vi "ADQUIRI_adq.vi"() -> ()   [LabVIEW 2019]
doc: "Programa que faz a leitura e a gravação em arquivo TXT de 13 canais provenientes da placa da National Instruments."
uses:
  <vilib>/DAQmx/read.llb/DAQmx Read (Analog 2D DBL NChan NSamp).vi
  <vilib>/Analysis/baseanly.llb/Mean (DBL).vi
  comunicacao.vi
  Aplicacao_atual_global_adq.vi
  <vilib>/DAQmx/configure/timing.llb/DAQmx Timing (Sample Clock).vi
  <vilib>/DAQmx/miscellaneous.llb/DAQmx Fill In Error Info.vi
  <vilib>/Utility/file.llb/Read Delimited Spreadsheet (string).vi
  <vilib>/Utility/file.llb/Write Delimited Spreadsheet (string).vi
  <vilib>/Analysis/NI_AALBase.lvlib
panel:
  out "P1-P2 VERDE":bool
  in  "pos_processamento":bool
  out "comunica funcionando":bool
  in  "Calibração":bool
  in  "COMUNICA":bool
  out "DAQmx Task Name":refnum<k21>
  in  "Visualizar":bool
  out "led viewing":bool
  out "Configuração":string
  in  "Pontos No Gráfico":dbl(knob)=497.5700948522667 scale=0.0..3000.0
  in  "Frequência":dbl=3000.0
  out "Ok":bool
  out "OK2":bool
  out "Ok R":bool
  out "OK2 R":bool
  out "SKM-AI-KF-COR":dbl
  out "SKM-FI-WF":dbl format="%#.2g"
  out "SKM-FIC-KF-COR":dbl format="%#.2g"
  in  "SAIR":bool
  out "JG(m/s)":dbl
  in  "TempoAquisicao":dbl=60.0
  out "JW(m/s)":dbl format="%#.6g"
  out "JK(m/s)":dbl format="%#.6g"
  out "Timer":i32 caption="Elapsed Time (s)"
  in  "COMEÇAR":bool
  out "Quantidade de\narquivos adquiridos":i64
  out "LED adquiri":bool
  out "Aquisição Automática":bool
  out "Linha de Teste":bool
  in  "Tab Control":enum32{"Gráfico", "Matriz"}(tab)
  out "retirando agua_indicador":bool
  in  "Retirando agua(?)":bool
  out "Aplicação":string
  in  "Help":bool
  out "Gráfico":dbl[][](graph)
  out "C1-M corrente":dbl format="%#_4g"
  out "C1-J corrente":dbl format="%#_4g"
  out "C2-M corrente":dbl format="%#_4g"
  out "C2-J corrente":dbl format="%#_4g"
  out "C3-M corrente":dbl format="%#_4g"
  out "C3-J corrente":dbl format="%#_4g"
  out "C4-M corrente":dbl format="%#_4g"
  out "C4-J corrente":dbl format="%#_4g"
  out "P1 corrente":dbl format="%#_4g"
  out "P2 corrente":dbl format="%#_4g"
  out "P3 corrente":dbl format="%#_4g"
  out "P4 corrente":dbl format="%#_4g"
  out "Pfundo corrente":dbl format="%#_4g"
  out "P4(kPa)":dbl format="%#.2g"
  out "P3(kPa)":dbl format="%#.2g"
  out "P2(kPa)":dbl format="%#.2g"
  out "P1(kPa)":dbl format="%#.2g"
  out "Pfundo(kPa)":dbl format="%#.2g"
  out "P4":dbl format="%#_2g"
  out "C4-J":dbl format="%#_2g"
  out "C4-M":dbl format="%#_2g"
  out "C3-J":dbl format="%#_2g"
  out "P3":dbl format="%#_2g"
  out "C3-M":dbl format="%#_2g"
  out "Pfundo":dbl format="%#_2g"
  out "C2-J":dbl format="%#_2g"
  out "P2":dbl format="%#_2g"
  out "C2-M":dbl format="%#_2g"
  out "P1":dbl format="%#_2g"
  out "C1-M":dbl format="%#_2g"
  out "C1-J":dbl format="%#_2g"
  out "Matriz":dbl[][](array[numeric])
  out "Finalizado":bool
  out "Aquisição":bool
  out "Visualização":bool
  out "Comunicação":bool
  in  "SIK-CV-001 2":bool
  in  "SIW-CV-001 2":bool
  in  "ValoresEnviados":T1
  out "SKS-NC-CV-006":bool
  in  "Valores":T2
  out "P1-P2 RED":bool
  out "P2-P3 RED":bool
  out "P3-P4 RED":bool
  out "P34/L [Pa/m]":dbl
  out "P23/L [Pa/m]":dbl
  out "P12/L [Pa/m]":dbl
  out "Valor Teórico[Pa/m]":dbl
  out "P3-P4 VERDE":bool
  out "P2-P3 VERDE":bool
  out "Valvulas":T3
  out "VALORES UDP":string[](array[string])
  out "reference out":refnum<vi>
  out "error out":errorcluster
  in  "SKM-AI-KF_CORIOLI [kg/m³]":dbl
  in  "SKM-FIC-KF_CORIOLI [kg/s]":dbl
  in  "SIW-CV-001":bool
  in  "SIK-CV-001":bool
  in  "Entrada - SKM-FI-WF [CLP]":dbl
  in  "Escala de Calibracao - SKM-FI-WF":cluster{"Escala Max":dbl, "Escala Min":dbl}
  # "m/s"
  # "<- Aquisição"
  # "[Hz]"
  # "Aquisição"
  # "[s]"
  # "m³/s"
  # "m/s"
  # "CHECK-UP"
  # "[s]"
  # "kg/s"
  # "P1, P3 & P4"
  # "m/s"
  # "kg/m³"
  # "P2"
  # "[mA]"
  # "[V]"
  # "[mA]"
  # "[V]"
  # "[mA]"
  # "[V]"
  # "[kPa]"
  # "[mA]"
  # "[V]"
  # "[mA]"
  # "[V]"
  # "[mA]"
  # "[V]"
  # "[kPa]"
  # "[mA]"
  # "[V]"
  # "[mA]"
  # "[V]"
  # "[mA]"
  # "[V]"
  # "[kPa]"
  # "[mA]"
  # "[V]"
  # "[mA]"
  # "[V]"
  # "[mA]"
  # "[V]"
  # "[kPa]"
  # "[mA]"
  # "[V]"
  # "[kPa]"
  # "MIN"
  # "MAX"
  # "P1"
  # "kPa"
  # "P2"
  # "kPa"
  # "P3"
  # "kPa"
  # "P4"
  # "kPa"
  # "Pfundo"
  # "kPa"
  # "Variáveis Selecionadas Para Aquisição"
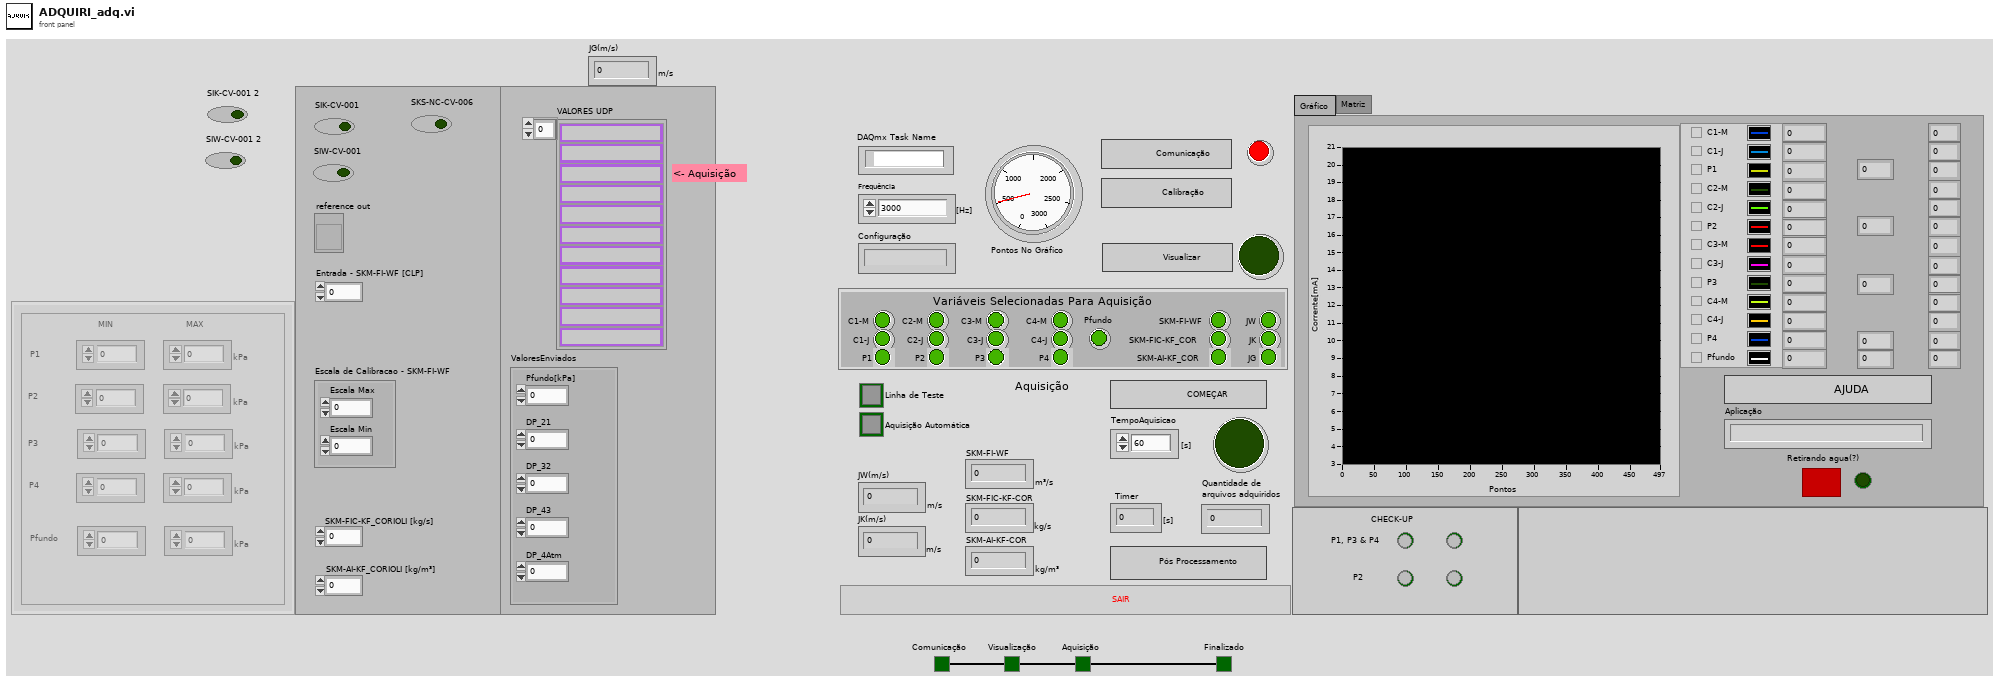
[diagram p1: front panel]
types:
  T1 = cluster{"Pfundo[kPa]":dbl, "DP_21":dbl, "DP_43":dbl, "DP_32":dbl, "DP_4Atm":dbl}
  T2 = cluster{"P1 MIN":i32, "P1 MAX":i32, "P2 MIN":i32, "P2 MAX":i32, "P3 MIN":i32, "P3 MAX":i32, "P4 MIN":i32, "P4 MAX":i32, "Pfu MIN":i32, "Pfu MAX":i32}
  T3 = cluster{"C1-M":bool, "C1-J":bool, "P1":bool, "C2-M":bool, "C2-J":bool, "P2":bool, "C3-M":bool, "C3-J":bool, "P3":bool, "C4-M":bool, "C4-J":bool, "P4":bool, "Pfundo":bool, "JW":bool, "JK":bool, "JG":bool, "SKM-FI-WF":bool, "SKM-FIC-KF_COR":bool, "SKM-AI-KF_COR":bool}
  T4 = enum8{"Enabled", "Disabled", "Disabled and Grayed Out"}
  T5 = enum32{"Invalid", "Standard", "Closed", "Hidden", "Minimized", "Maximized"}
  T6 = enum32{"Bad", "Idle", "Run top level", "Running"}
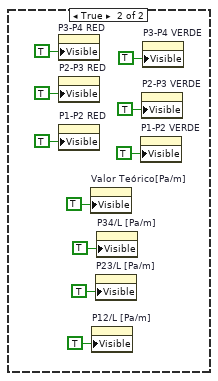
[diagram p3: hidden frame]
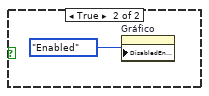
[diagram p5: hidden frame]
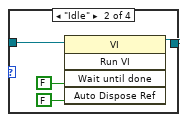
[diagram p6: hidden frame]
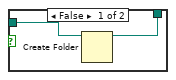
[diagram p9: hidden frame]
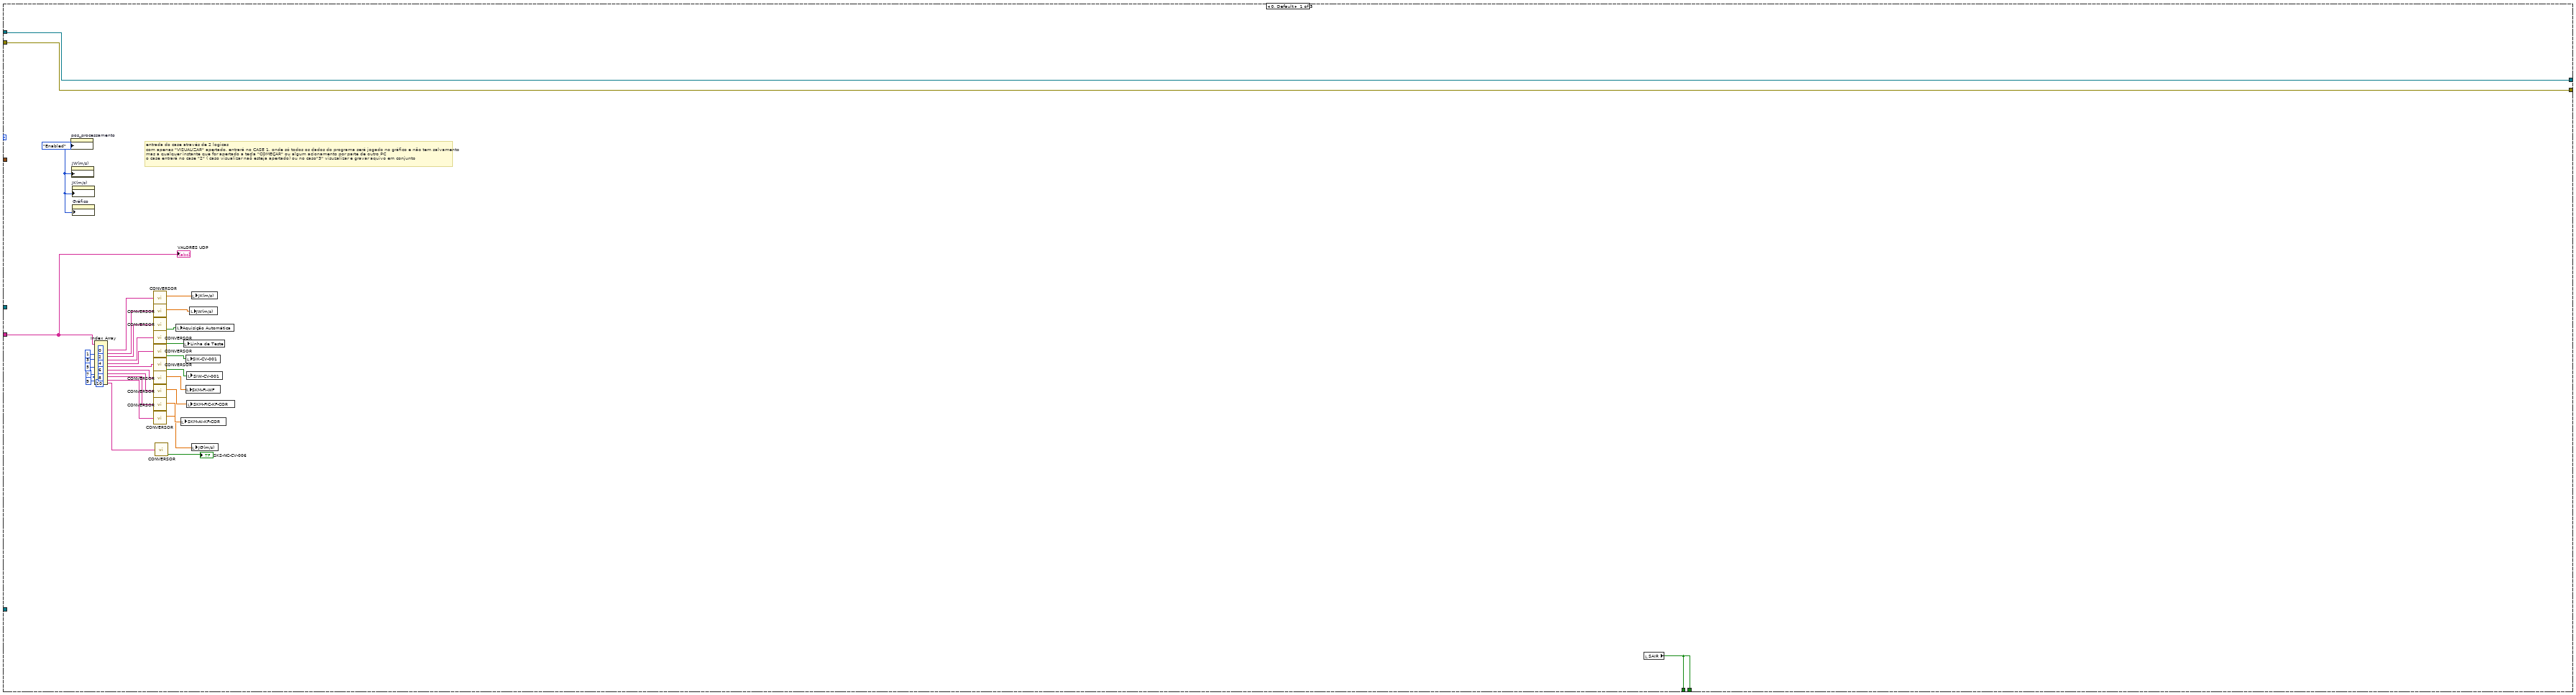
[diagram p11: hidden frame]
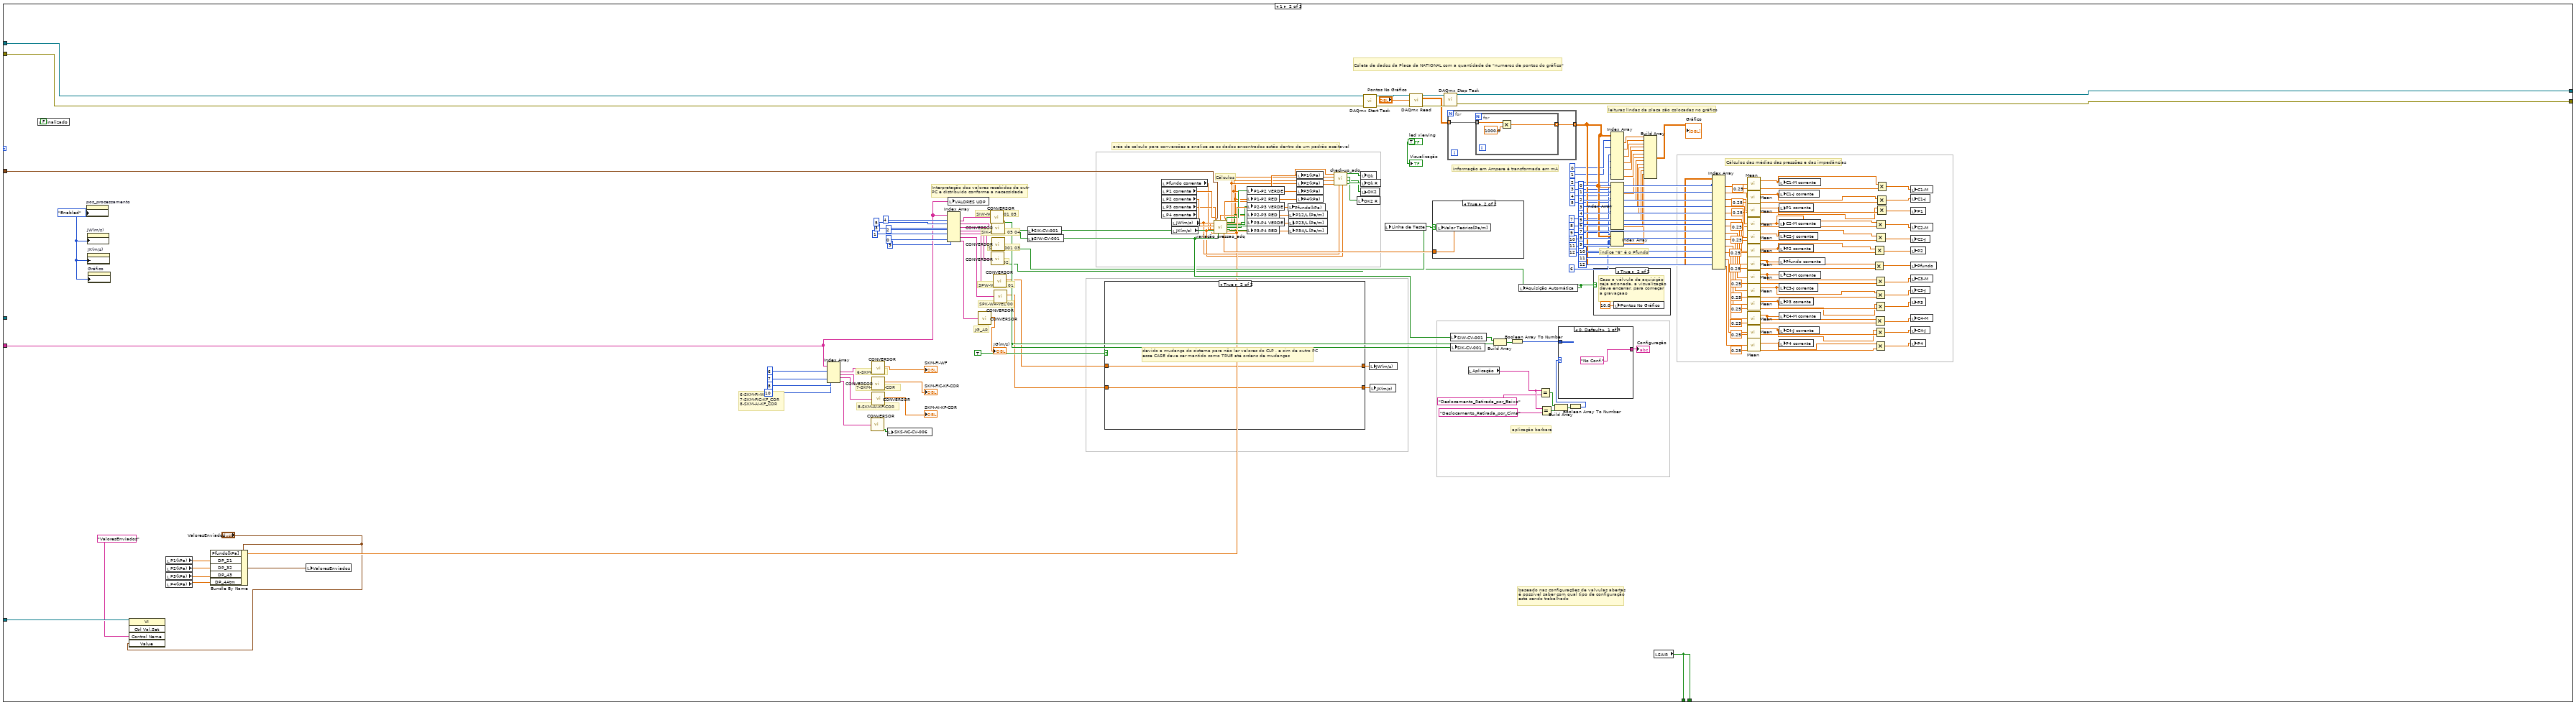
[diagram p12: hidden frame]
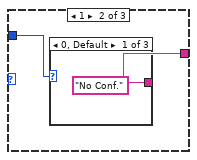
[diagram p13: hidden frame]
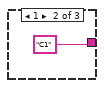
[diagram p14: hidden frame]
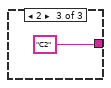
[diagram p15: hidden frame]
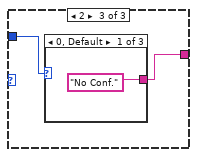
[diagram p16: hidden frame]
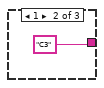
[diagram p17: hidden frame]
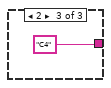
[diagram p18: hidden frame]
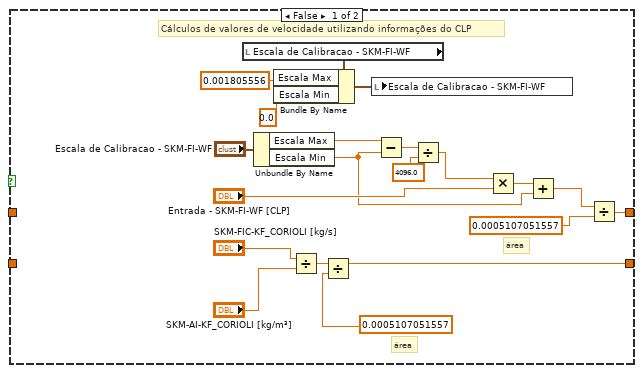
[diagram p19: hidden frame]
diagram:
  # "Abre a VI"
  n1 = property class="VI"("Front Panel.Open"=TRUE ("Front Panel Window:Open")) -> (error out=w1:errorcluster)  [unwired: 2 in, 1 out]
  n2 = flat-sequence {
    tunnel: [w5] -> w3
    tunnel: w1 -> [w4]
    tunnel: w3 -> [w806]
    frame #0 {
      n3 = while {
        shift-right: [w8] -> w5
        shift-left: w4 -> [w7]
        stop <- w6 stop-if-true
        # "Loop responsável\npor manter o \nadquiri rodando\n\nmesmo após uma \naquisição ou \nvisualização dos \ndados\no adquiri não irá\nfechar, e irá \naguardar um novo\ncomando"
        n4 = stacked-sequence {
          tunnel: [w29 _ _ _] -> w8
          tunnel: w7 -> [w29 _ _ _]
          tunnel: [_ _ _ w799] -> w6
          frame #0 {
            w20 = FALSE ("Visualisa")
            w9 = FALSE ("Visualisa")
            w33 = 0.0 ("element")
            # "aplicação barbara"
            # "Nessa parte do cógido, procuramos na aplicação atual, o seu diretório de armazenamento de dados, chamado\n\"DADOS\", cria-o se o mesmo n existir, caso exista, irá retornar a quantidade de arquivos ja adquiridos"
            # "Vi lê as configurações já definidas da aplicação atual e coloca na vairável\n\"VALVULAS\" para facilitar o manuzeio nesse programa"
            # "nessa parte do código , para o ADQUIRI teer acesso a algumas informações do CLP\no computador ADQUIRI evita de comunicar com o CLP para evitar erros futuros, então ele\npega as informações do computador SuperTorre, que é responsável por tratar esses dados\nnessa parte do código, procuramos o diretório UDP e colocamos para rodar o programa\n\"CLIENTE GERAL\" que será responsável por receber as informações do outro PC que contém\no programa\" SERVER GERAL\""
            # "Primeria parte da sequencia  do adquiri, inicia com todas as \nconfigurações e controle em seus estados default\nmatriz de armazenamento com até 17 posições para \narmazenamento de dados e transcrissão para o arquivo txt \nno final da sequencia\npontos no grafico com visualização de 3000 pontos por \nsegundo\ntempo de aquisição inicializado em 30 segundos, mas pode \nser alterado conforme a preferÊncia do usuário\nTimer inicia em 0, que será o tempo atual de aquisição\na configuração da aplicação inicia em default , pois ao longo \ndos acionamento do supervisório, irá saber de qual \nconfiguração se trata\ncontrole de pontos no gráfico encontra ativado\n\nem verde, temos todos os booleanos que necessitam ser\ninicializados em FALSE"
            # "Variáveis que precisam começar com valores iniciais"
            # "indicadores que precisam iniciar desligados"
            n5 = global read "Aplicacao_atual_global_adq.vi" "APLICACAO ATUAL"() -> (w10:string)
            "Aplicação" <- w10
            n6 = flat-sequence {
              frame #0 {
                n7 = global read "comunicacao.vi" "comunicacao"() -> (w55:bool)
                n8 = case shown="False" w55 {
                  frame False {
                    n9 = while {
                      stop <- w56 stop-if-true
                      n10 = One Button Dialog(message="LIGUE O SERVER E \nAPÓS ISSO,\n LIGAR COMUNICAÇÃO", button name ("OK")="OK") -> (true=w56:bool)
                    }
                  }
                  frame True {
                  }
                }
              }
              frame #1 {
                n11 = global read "comunicacao.vi" "comunicacao"() -> (w59:bool)
                n12 = case shown="False" w59 {
                  frame False {
                    n13 = while {
                      stop <- "COMUNICA" stop-if-true
                      n14 = property on="Gráfico" class="WFGraph (strict)"("DisabledEnum"=T4."Disabled and Grayed Out" ("Disabled")) -> ()  [unwired: 2 in, 2 out]
                    }
                  }
                  frame True {
                    n15 = property on="Gráfico" class="WFGraph (strict)"("DisabledEnum"=T4."Enabled" ("Disabled")) -> ()  [unwired: 2 in, 2 out]
                  }
                }
              }
              frame #2 {
                n16 = Current VI's Path() -> (path=w68:path)
                n17 = Strip Path(path=w68) -> (stripped path=w69:path)  [unwired: 1 out]
                n18 = Strip Path(path=w69) -> (stripped path=w70:path)  [unwired: 1 out]
                n19 = Build Path(base path=w70, name or relative path="UDP\\CLIENTE GERAL.vi") -> (appended path=w71:path)
                n20 = Open VI Reference(vi path=w71) -> (vi reference=w64:refnum<vi>)  [unwired: 5 in, 1 out]
                n21 = property class="VI"(reference=w64) -> (reference out=w65:refnum<vi>, "Exec.State"=w66:T6)  [unwired: 1 in, 1 out]
                n22 = case shown="\"Bad\", Default" w66 {
                  tunnel: w65 -> [w72 w74 w77 w78]
                  tunnel: [w72 w73 w77 w78] -> w63
                  frame "Bad", Default {
                  }
                  frame "Idle" {
                    n23 = invoke class="VI" method="Run VI"(reference=w74, "Wait until done"=FALSE ("Wait Until Done"), "Auto Dispose Ref"=FALSE ("Auto Dispose Reference")) -> (reference out=w73:refnum<vi>)  [unwired: 2 in, 4 out]
                  }
                  frame "Run top level" {
                  }
                  frame "Running" {
                  }
                }
                "reference out" <- w63
              }
            }
            n24 = Current VI's Path() -> (path=w28:path)
            n25 = Strip Path(path=w28) -> (stripped path=w27:path)  [unwired: 1 out]
            n26 = Equal?(x=w10, y="Deslocamento_Retirada_por_Baixo") -> (x = y?=w17:bool)
            n27 = Equal?(x=w10, y="Deslocamento_Retirada_por_Cima") -> (x = y?=w16:bool)
            n28 = Or(x=w17, y=w16) -> (x .or. y?=w15:bool)
            n29 = Build Path(base path=w27, name or relative path="PosProcessamento_UDP_NI\\data") -> (appended path=w23:path)
            n30 = property on="Pontos No Gráfico" class="Knob (strict)"("DisabledEnum"=T4."Enabled" ("Disabled")) -> ()  [unwired: 2 in, 2 out]
            n31 = property on="Calibração" class="Bool (strict)"("DisabledEnum"=T4."Enabled" ("Disabled")) -> ()  [unwired: 2 in, 2 out]
            n32 = Initialize Array(w33, w33, 16.0 ("element")) -> (→"Matriz":dbl[][])
            n33 = local write "Configuração"("No Conf." ("Configuration")) -> ()
            n34 = case shown="False" w15 {
              frame False {
                n35 = property on="P3-P4 RED" class="Bool (strict)"("Visible"=FALSE) -> ()  [unwired: 2 in, 2 out]
                n36 = property on="P2-P3 RED" class="Bool (strict)"("Visible"=FALSE) -> ()  [unwired: 2 in, 2 out]
                n37 = property on="P1-P2 RED" class="Bool (strict)"("Visible"=FALSE) -> ()  [unwired: 2 in, 2 out]
                n38 = property on="P1-P2 VERDE" class="Bool (strict)"("Visible"=FALSE) -> ()  [unwired: 2 in, 2 out]
                n39 = property on="P2-P3 VERDE" class="Bool (strict)"("Visible"=FALSE) -> ()  [unwired: 2 in, 2 out]
                n40 = property on="P3-P4 VERDE" class="Bool (strict)"("Visible"=FALSE) -> ()  [unwired: 2 in, 2 out]
                n41 = property on="P12/L [Pa/m]" class="DigNum (strict)"("Visible"=FALSE) -> ()  [unwired: 2 in, 2 out]
                n42 = property on="P23/L [Pa/m]" class="DigNum (strict)"("Visible"=FALSE) -> ()  [unwired: 2 in, 2 out]
                n43 = property on="P34/L [Pa/m]" class="DigNum (strict)"("Visible"=FALSE) -> ()  [unwired: 2 in, 2 out]
                n44 = property on="Valor Teórico[Pa/m]" class="DigNum (strict)"("Visible"=FALSE) -> ()  [unwired: 2 in, 2 out]
              }
              frame True {
                n45 = property on="P3-P4 RED" class="Bool (strict)"("Visible"=TRUE) -> ()  [unwired: 2 in, 2 out]
                n46 = property on="P2-P3 RED" class="Bool (strict)"("Visible"=TRUE) -> ()  [unwired: 2 in, 2 out]
                n47 = property on="P1-P2 RED" class="Bool (strict)"("Visible"=TRUE) -> ()  [unwired: 2 in, 2 out]
                n48 = property on="Valor Teórico[Pa/m]" class="DigNum (strict)"("Visible"=TRUE) -> ()  [unwired: 2 in, 2 out]
                n49 = property on="P12/L [Pa/m]" class="DigNum (strict)"("Visible"=TRUE) -> ()  [unwired: 2 in, 2 out]
                n50 = property on="P23/L [Pa/m]" class="DigNum (strict)"("Visible"=TRUE) -> ()  [unwired: 2 in, 2 out]
                n51 = property on="P34/L [Pa/m]" class="DigNum (strict)"("Visible"=TRUE) -> ()  [unwired: 2 in, 2 out]
                n52 = property on="P1-P2 VERDE" class="Bool (strict)"("Visible"=TRUE) -> ()  [unwired: 2 in, 2 out]
                n53 = property on="P2-P3 VERDE" class="Bool (strict)"("Visible"=TRUE) -> ()  [unwired: 2 in, 2 out]
                n54 = property on="P3-P4 VERDE" class="Bool (strict)"("Visible"=TRUE) -> ()  [unwired: 2 in, 2 out]
              }
            }
            n55 = local write "Timer"(0.0 ("Timer")) -> ()
            n56 = call <vilib>:"Check if File or Folder Exists.vi"("path"=w23) -> ("file or folder exists?"=w26:bool, "dup path"=w25:path)  [unwired: 8 in, 1 out]
            n57 = case shown="True" w26 {
              tunnel: w25 -> [w80 w81]
              tunnel: [w79 w81] -> w24
              frame False {
                n58 = Create Folder(path (use dialog)=w80) -> (created path=w79:path)  [unwired: 2 in, 2 out]
              }
              frame True {
              }
            }
            n59 = File/Directory Info(path=w24) -> (size=w13:i64)  [unwired: 1 in, 6 out]
            n60 = local write "Visualização"(w9) -> ()
            n61 = local write "led viewing"(w9) -> ()
            n62 = local write "LED adquiri"(w9) -> ()
            n63 = local write "Visualizar"(w9) -> ()
            n64 = local write "P1-P2 VERDE"(w9) -> ()
            n65 = local write "P1-P2 RED"(w9) -> ()
            n66 = local write "P2-P3 VERDE"(w9) -> ()
            n67 = local write "P2-P3 RED"(w9) -> ()
            n68 = local write "P3-P4 VERDE"(w9) -> ()
            n69 = local write "P3-P4 RED"(w9) -> ()
            n70 = local write "COMEÇAR"(w9) -> ()
            n71 = local write "Help"(w9) -> ()
            n72 = local write "SAIR"(w9) -> ()
            n73 = local write "Aquisição Automática"(w9) -> ()
            n74 = local write "comunica funcionando"(w9) -> ()
            n75 = local write "Comunicação"(w9) -> ()
            n76 = local write "Aquisição"(w9) -> ()
            n77 = Decrement(x=w13) -> (x-1=→"Quantidade de\narquivos adquiridos":i64)
            n78 = local write "Ok"(w20) -> ()
            n79 = local write "Ok R"(w20) -> ()
            n80 = local write "OK2"(w20) -> ()
            n81 = local write "OK2 R"(w20) -> ()
            n82 = call "leitura_configuracao_valvulas_adq.vi"() -> ("Valvulas"=→"Valvulas":T3)  [unwired: 6 in]
          }
          frame #1 {
            # "nessa etapa do programa, pegamos as referências dessas Vi\n\"LEITURA VALORES CLIENTE\" E \"CLIENTE GERAL\" que JÁ ESTÃO\nRODANDO EM OFF\ncom as refências em mãos, iremos jagá-las para dentro do loop"
            n83 = Current VI's Path() -> (path=w96:path)
            n84 = Current VI's Path() -> (path=w107:path)
            n85 = Strip Path(path=w107) -> (stripped path=w108:path)  [unwired: 1 out]
            n86 = Strip Path(path=w96) -> (stripped path=w90:path)  [unwired: 1 out]
            n87 = Strip Path(path=w108) -> (stripped path=w85:path)  [unwired: 1 out]
            n88 = Build Path(base path=w90, name or relative path="calibracao_adq.vi") -> (appended path=w94:path)
            n89 = Build Path(base path=w85, name or relative path="UDP\\ENVIA VALORES-CLIENTE.vi") -> (appended path=w84:path)
            n90 = Build Path(base path=w85, name or relative path="UDP\\LEITURA VALORES CLIENTE.vi") -> (appended path=w109:path)
            n91 = Build Path(base path=w85, name or relative path="UDP\\CLIENTE GERAL.vi") -> (appended path=w104:path)
            n92 = Open VI Reference(vi path=w84) -> (vi reference=w82:refnum<vi>)  [unwired: 5 in, 1 out]
            n93 = Open VI Reference(vi path=w94, error in (no error)=errorcluster {"status"=FALSE, "code"=0, "source"=""}) -> (vi reference=w93:refnum<vi>, error out=w92:errorcluster)  [unwired: 4 in]
            n94 = Open VI Reference(vi path=w109) -> (vi reference=w105:refnum<vi>)  [unwired: 5 in, 1 out]
            n95 = Open VI Reference(vi path=w104) -> (vi reference=w102:refnum<vi>)  [unwired: 5 in, 1 out]
            n96 = invoke class="VI" method="Run VI"(reference=w93, error in=w92, "Wait until done"=FALSE ("Wait Until Done"), "Auto Dispose Ref"=TRUE ("Auto Dispose Reference")) -> (reference out=w98:refnum<vi>, error out=w97:errorcluster)  [unwired: 1 in, 3 out]
            n97 = invoke class="VI" method="Ctrl Val.Get"(reference=w98, error in=w97, "Control Name"="Valores") -> (reference out=w88:refnum<vi>, error out=w87:errorcluster, "Get Control Value Variant"=w86:variant)  [unwired: 1 in, 1 out]
            n98 = while {
              tunnel: w105 -> [w123]
              tunnel: w102 -> [w146]
              shift-right: [w136] -> w89
              shift-left: w88 -> [w132]
              shift-right: [w135] -> _
              shift-left: w87 -> [w133]
              shift-right: [w131] -> _
              shift-left: w86 -> [w134]
              tunnel: w82 -> [w124]
              stop <- w159 stop-if-true
              w121 = refnum<k21> "ADQUIRE" ("DAQmx Task Name")
              w120 = 10123 items=["Finite Samples"=10178, "Continuous Samples"=10123, "Hardware Timed Single Point"=12522] ("sample mode")
              w111 = FALSE ("visu led")
              # "Parte de comunicação com a placa da NATIONAL\nINSTRUMENTS\nno módulo de comunicação chamado DAQmx\nselecionamos o tipo \"continuous SAMPLES\" para a\ncoleta de amostras contínuas\ntambém entramos com o nome de TASK chamado\nADQUIRE, que já contém informações de leitura \njá pré programadas\nFrequência padrão de 3000Hz"
              # "10"
              # "9"
              # "8"
              # "7"
              # "6"
              # "5"
              # "4"
              # "3"
              # "2"
              # "1"
              # "0"
              # "acionamento automático recebido de outro\nPC"
              # "Default dos botões"
              # "Caso as configurações não desejam\nincluir alguma velocidade na aquisição\na mesma será desabilitada"
              # "Coleta os valores das variáveis enviadas abaixo\nos valores são devolvidos na mesma ordem"
              # "Envia para o programa de comunicação com o outro computador\numa lista de nomes de variáveis que o ADQUIRE nessecita \nos nomes precisam ser enviados em array de STRING para o funcionamento\ndo programa de comunicação."
              # "ADQ 02"
              n99 = local read "Valvulas"() -> (w150:T3)
              n100 = local write "Ok R"(w111) -> ()
              n101 = local write "Visualização"(w111) -> ()
              n102 = local write "led viewing"(w111) -> ()
              n103 = local write "OK2"(w111) -> ()
              n104 = local write "OK2 R"(w111) -> ()
              n105 = local write "Ok"(w111) -> ()
              n106 = case shown="True" "Help" {
                frame False {
                  # "Botão Help destinado a abrir documentos e pesquisas relacionadas\nele também abre uma janela explicando sucintamente o objetivo do \nprograma ADQUIRE"
                }
                frame True {
                  n107 = stacked-sequence {
                    frame #0 {
                      n108 = Current VI's Path() -> (path=w741:path)
                      n109 = Current VI's Path() -> (path=w735:path)
                      n110 = Strip Path(path=w741) -> (stripped path=w740:path)  [unwired: 1 out]
                      n111 = Strip Path(path=w735) -> (stripped path=w734:path)  [unwired: 1 out]
                      n112 = Build Path(base path=w740, name or relative path="Help_difinicao_adq.vi") -> (appended path=w738:path)
                      n113 = Build Path(base path=w734, name or relative path="help_pdfs_adq.vi") -> (appended path=w732:path)
                      n114 = Open VI Reference(vi path=w738) -> (vi reference=w745:refnum<vi>, error out=w744:errorcluster)  [unwired: 5 in]
                      n115 = Open VI Reference(vi path=w732) -> (vi reference=w743:refnum<vi>, error out=w742:errorcluster)  [unwired: 5 in]
                      n116 = invoke class="VI" method="Run VI"(reference=w745, error in=w744, "Wait until done"=FALSE ("Wait Until Done"), "Auto Dispose Ref"=FALSE ("Auto Dispose Reference")) -> ()  [unwired: 1 in, 5 out]
                      n117 = invoke class="VI" method="Run VI"(reference=w743, error in=w742, "Wait until done"=FALSE ("Wait Until Done"), "Auto Dispose Ref"=FALSE ("Auto Dispose Reference")) -> ()  [unwired: 1 in, 5 out]
                    }
                    frame #1 {
                      n118 = local write "Help"(FALSE ("Help")) -> ()
                    }
                  }
                }
              }
              n119 = Unbundle By Name(w150) -> ("JW"=w151:bool, "JK"=w152:bool, "JG"=w153:bool)
              n120 = case shown="True" w151 {
                frame False {
                  n121 = property on="JW(m/s)" class="DigNum (strict)"("DisabledEnum"=T4."Disabled and Grayed Out" ("Disabled")) -> ()  [unwired: 2 in, 2 out]
                }
                frame True {
                  n122 = property on="JW(m/s)" class="DigNum (strict)"("DisabledEnum"=T4."Enabled" ("Disabled")) -> ()  [unwired: 2 in, 2 out]
                }
              }
              n123 = case shown="True" w152 {
                frame False {
                  n124 = property on="JK(m/s)" class="DigNum (strict)"("DisabledEnum"=T4."Disabled and Grayed Out" ("Disabled")) -> ()  [unwired: 2 in, 2 out]
                }
                frame True {
                  n125 = property on="JK(m/s)" class="DigNum (strict)"("DisabledEnum"=T4."Enabled" ("Disabled")) -> ()  [unwired: 2 in, 2 out]
                }
              }
              n126 = case shown="True" w153 {
                frame False {
                  n127 = property on="JG(m/s)" class="DigNum (strict)"("DisabledEnum"=T4."Disabled and Grayed Out" ("Disabled")) -> ()  [unwired: 2 in, 2 out]
                }
                frame True {
                  n128 = property on="JG(m/s)" class="DigNum (strict)"("DisabledEnum"=T4."Enabled" ("Disabled")) -> ()  [unwired: 2 in, 2 out]
                }
              }
              n129 = case shown="False" "Calibração" {
                tunnel: [w705 w713] -> w136
                tunnel: [w706 w712] -> w135
                tunnel: [w707 w711] -> w131
                tunnel: w132 -> [w704 w710]
                tunnel: w133 -> [w703 w709]
                tunnel: w134 -> [_ _]
                frame False {
                  n130 = invoke class="VI" method="Ctrl Val.Get"(reference=w704, error in=w703, "Control Name"="Valores") -> (reference out=w705:refnum<vi>, error out=w706:errorcluster, "Get Control Value Variant"=w707:variant)  [unwired: 1 in, 1 out]
                }
                frame True {
                  n131 = stacked-sequence {
                    tunnel: [w718 _] -> w713
                    tunnel: [w717 _] -> w712
                    tunnel: [w716 _] -> w711
                    tunnel: w710 -> [w715 _]
                    tunnel: w709 -> [w714 _]
                    frame #0 {
                      n132 = invoke class="VI" method="FP.Open"(reference=w715, error in=w714, "State"=T5."Standard") -> (reference out=w720:refnum<vi>, error out=w719:errorcluster)  [unwired: 2 in, 3 out]
                      n133 = invoke class="VI" method="Ctrl Val.Get"(reference=w720, error in=w719, "Control Name"="Valores") -> (reference out=w718:refnum<vi>, error out=w717:errorcluster, "Get Control Value Variant"=w716:variant)  [unwired: 1 in, 1 out]
                    }
                    frame #1 {
                      n134 = local write "Calibração"(FALSE ("Calibração")) -> ()
                    }
                  }
                }
              }
              n135 = invoke class="VI" method="Ctrl Val.Get"(reference=w123, "Control Name"="VALORES") -> ("Get Control Value Variant"=w149:variant)  [unwired: 2 in, 3 out]
              n136 = property on="Gráfico" class="WFGraph (strict)"("DisabledEnum"=T4."Enabled" ("Disabled")) -> ()  [unwired: 2 in, 2 out]
              n137 = Variant To Data(type=string[] [] ("Array"), Variant=w149) -> (data=w128:string[])  [unwired: 1 in, 1 out]
              n138 = To Variant(anything=string[] ["JK", "JW", "ADQ", "SIT-NC-CV-001", "SIK-NC-CV-001", "SIW-NC-CV-001", "SKM-FI-WF", "SKM-FIC-KF_COR", "SKM-AI-KF_COR", "JG", "SKS-NC-CV-006"] ("NOMES")) -> (Variant=w141:variant)
              n139 = case shown="True" "pos_processamento" {
                frame False {
                }
                frame True {
                  n140 = Current VI's Path() -> (path=w169:path)
                  n141 = Strip Path(path=w169) -> (stripped path=w170:path)  [unwired: 1 out]
                  n142 = Build Path(base path=w170, name or relative path="PosProcessamento_UDP_NI\\main_PosProcessamento_UDP_NI.vi") -> (appended path=w171:path)
                  n143 = Open VI Reference(vi path=w171) -> (vi reference=w162:refnum<vi>)  [unwired: 5 in, 1 out]
                  n144 = invoke class="VI" method="FP.Open"(reference=w162, "Activate"=TRUE ("Activate?"), "State"=T5."Standard") -> (reference out=w165:refnum<vi>)  [unwired: 2 in, 4 out]
                  n145 = invoke class="VI" method="Run VI"(reference=w165, "Wait until done"=FALSE ("Wait Until Done")) -> (reference out=w166:refnum<vi>)  [unwired: 3 in, 4 out]
                  n146 = Close Reference(reference=w166) -> ()  [unwired: 1 in, 1 out]
                }
              }
              n147 = invoke class="VI" method="Ctrl Val.Set"(reference=w146, "Control Name"="NOMES", "Value"=w141) -> ()  [unwired: 2 in, 5 out]
              n148 = Index Array(array=w128, index=2) -> (element=w144:string)
              n149 = call "CONVERSOR.vi"("String"=w144) -> ("boolean"=w143:bool)  [unwired: 6 in, 3 out]
              "Aquisição Automática" <- w143
              n150 = Not Equal?(x=w128, y="") -> (x != y?=w127:bool[])
              n151 = Get Variant Attribute(Variant=w131, name="Valores") -> ()  [unwired: 2 in, 4 out]
              n152 = Variant To Data(type="Valores", Variant=w131) -> (data=w129:T2)  [unwired: 1 in, 1 out]
              n153 = Index Array(array=w127, index=0) -> (element=→"comunica funcionando" →"Comunicação":bool)
              n154 = local write "Valores"(w129) -> ()
              n155 = Or(x="COMEÇAR", y=w143) -> (x .or. y?=w156:bool)
              n156 = Build Array("Visualizar", w156) -> (w161:bool[])
              n157 = Boolean Array To Number(Boolean array=w161) -> (number=w160:u32)
              n158 = call-poly <vilib>:"DAQmx Timing.vi"("task/channels in"=w121, "sample mode"=w120, "rate"="Frequência", "source"=tag "OnboardClock") -> ("task out"=w118:refnum<k21>, "error out"=w117:errorcluster)  [unwired: 10 in]
              n159 = case shown="2, 3" w160 {
                tunnel: [w173 w239 w449] -> w158
                tunnel: [w173 w239 w448] -> w157
                tunnel: w128 -> [w207 w313 w447]
                tunnel: w118 -> [w209 w303 _]
                tunnel: w117 -> [w208 w302 _]
                tunnel: [w209 w301 w443] -> w115
                tunnel: [w208 w300 w444] -> w114
                tunnel: w129 -> [_ w257 w446]
                tunnel: w124 -> [_ w244 w445]
                tunnel: w123 -> [_ _ w442]
                frame 0, Default {
                  w172 = T4."Enabled" ("Disabled")
                  # "entrada do case através de 2 logicas\ncom apenas \"VISUALIZAR\" apertado, entrará no CASE 1, onde só todos os dados do programa será jogado no gráfico e não tem salvamento\nmas a qualquer instante que for apertado a tecla \"COMEÇAR\" ou algum acionamento por parte de outro PC\no case entrará no case \"2\" ( caso visualizar naõ esteja apertado) ou no caso\"3\" visuzalizar e gravar aquivo em conjunto"
                  n160 = property on="pos_processamento" class="Bool"("DisabledEnum"=w172) -> ()  [unwired: 2 in, 2 out]
                  n161 = property on="JW(m/s)" class="DigNum (strict)"("DisabledEnum"=w172) -> ()  [unwired: 2 in, 2 out]
                  n162 = property on="JK(m/s)" class="DigNum (strict)"("DisabledEnum"=w172) -> ()  [unwired: 2 in, 2 out]
                  n163 = property on="Gráfico" class="WFGraph (strict)"("DisabledEnum"=w172) -> ()  [unwired: 2 in, 2 out]
                  n164 = Index Array(array=w207, index #1=0 ("index"), index #2=1 ("index"), index #3=2 ("index"), index #4=3 ("index"), index #5=4 ("index"), index #6=5 ("index"), index #7=6 ("index"), index #8=7 ("index"), index #9=8 ("index"), index #10=9 ("index"), index #11=10 ("index")) -> (element #1=w196:string, element #2=w195:string, element #3=w194:string, element #4=w193:string, element #5=w192:string, element #6=w191:string, element #7=w190:string, element #8=w189:string, element #9=w188:string, element #10=w187:string, element #11=w176:string)
                  n165 = call "CONVERSOR.vi"("String"=w196) -> ("float"=w186:dbl)  [unwired: 6 in, 3 out]
                  n166 = call "CONVERSOR.vi"("String"=w195) -> ("float"=w185:dbl)  [unwired: 6 in, 3 out]
                  n167 = call "CONVERSOR.vi"("String"=w194) -> ("boolean"=w184:bool)  [unwired: 6 in, 3 out]
                  n168 = call "CONVERSOR.vi"("String"=w193) -> ("boolean"=w183:bool)  [unwired: 6 in, 3 out]
                  n169 = call "CONVERSOR.vi"("String"=w192) -> ("boolean"=w182:bool)  [unwired: 6 in, 3 out]
                  n170 = call "CONVERSOR.vi"("String"=w191) -> ("boolean"=w181:bool)  [unwired: 6 in, 3 out]
                  n171 = call "CONVERSOR.vi"("String"=w190) -> ("float"=w180:dbl)  [unwired: 6 in, 3 out]
                  n172 = call "CONVERSOR.vi"("String"=w189) -> ("float"=w179:dbl)  [unwired: 6 in, 3 out]
                  n173 = call "CONVERSOR.vi"("String"=w188) -> ("float"=w178:dbl)  [unwired: 6 in, 3 out]
                  n174 = call "CONVERSOR.vi"("String"=w187) -> ("float"=w177:dbl)  [unwired: 6 in, 3 out]
                  n175 = call "CONVERSOR.vi"("String"=w176) -> ("boolean"=→"SKS-NC-CV-006":bool)  [unwired: 6 in, 3 out]
                  n176 = local write "Aquisição Automática"(w184) -> ()
                  n177 = local write "SKM-AI-KF-COR"(w178) -> ()
                  n178 = local write "Linha de Teste"(w183) -> ()
                  n179 = local write "SKM-FI-WF"(w180) -> ()
                  n180 = local write "SIK-CV-001"(w182) -> ()
                  n181 = local write "SIW-CV-001"(w181) -> ()
                  n182 = local write "SKM-FIC-KF-COR"(w179) -> ()
                  n183 = local write "JW(m/s)"(w185) -> ()
                  n184 = local write "JK(m/s)"(w186) -> ()
                  n185 = local write "JG(m/s)"(w177) -> ()
                  n186 = local read "SAIR"() -> (w173:bool)
                  "VALORES UDP" <- w207
                }
                frame 1 {
                  w238 = T4."Enabled" ("Disabled")
                  w241 = TRUE ("visu led")
                  # "Cálculos"
                  # "aplicação barbara"
                  # "JG_AR"
                  # "6-SKM-FI-WF"
                  # "7-SKM-FIC-KF-COR"
                  # "8-SKM-AI-KF-COR"
                  # "6-SKM-FI-WF\n7-SKM-FIC-KF_COR\n8-SKM-AI-KF_COR"
                  # "indice \"6\" é o Pfundo"
                  # "leituras lindas da placa são colocadas no gráfico"
                  # "baseado nas configurações de valvulas abertas\né possível saber com qual tipo de configuração \nestá sendo trabalhado"
                  # "aréa de calculo para conversões e analise se os dados encontrados estão dentro de um padrão aceitavel"
                  # "Interpretação dos valores recebidos de outr\nPC e distribuido conforme a necessidade"
                  # "informação em Ampere é transformada em mA"
                  # "Coleta de dados da Placa da NATIONAL com a quantidade de \"numeros de pontos do gráfico\""
                  # "ADQ 02"
                  # "SIW-NC-CV-001 05"
                  # "SIK-CV-001 05 04"
                  # "SIT-CV-001 03"
                  # "SPW-WR-VEL 01"
                  # "SPK-WR-VEL 00"
                  # "Cálculos das médias das pressões e das impedâncias"
                  n187 = local write "Finalizado"(FALSE ("Finalizado")) -> ()
                  n188 = property on="pos_processamento" class="Bool"("DisabledEnum"=w238) -> ()  [unwired: 2 in, 2 out]
                  n189 = property on="JW(m/s)" class="DigNum (strict)"("DisabledEnum"=w238) -> ()  [unwired: 2 in, 2 out]
                  n190 = property on="JK(m/s)" class="DigNum (strict)"("DisabledEnum"=w238) -> ()  [unwired: 2 in, 2 out]
                  n191 = property on="Gráfico" class="WFGraph (strict)"("DisabledEnum"=w238) -> ()  [unwired: 2 in, 2 out]
                  n192 = invoke class="VI" method="Ctrl Val.Set"(reference=w244, "Control Name"="ValoresEnviados", "Value"="ValoresEnviados") -> ()  [unwired: 2 in, 5 out]
                  n193 = local read "P1(kPa)"() -> (w213:dbl)
                  n194 = local read "P2(kPa)"() -> (w212:dbl)
                  n195 = local read "P3(kPa)"() -> (w211:dbl)
                  n196 = local read "P4(kPa)"() -> (w210:dbl)
                  n197 = Index Array(array=w313, index #1=6 ("index"), index #2=7 ("index"), index #3=8 ("index"), index #4=10 ("index")) -> (element #1=w309:string, element #2=w308:string, element #3=w307:string, element #4=w255:string)
                  n198 = call "CONVERSOR.vi"("String"=w255) -> ("boolean"=w254:bool)  [unwired: 6 in, 3 out]
                  n199 = call "CONVERSOR.vi"("String"=w308) -> ("float"=→"SKM-FIC-KF-COR":dbl)  [unwired: 6 in, 3 out]
                  n200 = call "CONVERSOR.vi"("String"=w309) -> ("float"=→"SKM-FI-WF":dbl)  [unwired: 6 in, 3 out]
                  n201 = call "CONVERSOR.vi"("String"=w307) -> ("float"=→"SKM-AI-KF-COR":dbl)  [unwired: 6 in, 3 out]
                  n202 = local write "SKS-NC-CV-006"(w254) -> ()
                  n203 = Index Array(array=w313, index #1=4 ("index"), index #2=5 ("index"), index #3=3 ("index"), index #4=2 ("index"), index #5=1 ("index"), index #6=0 ("index"), index #7=9 ("index")) -> (element #1=w330:string, element #2=w329:string, element #3=w326:string, element #4=w322:string, element #5=w318:string, element #6=w315:string, element #7=w298:string)
                  n204 = local write "VALORES UDP"(w313) -> ()
                  n205 = call "CONVERSOR.vi"("String"=w298) -> ("float"=→"JG(m/s)":dbl)  [unwired: 6 in, 3 out]
                  n206 = call "CONVERSOR.vi"("String"=w330) -> ("boolean"=w324:bool)  [unwired: 6 in, 3 out]
                  n207 = call "CONVERSOR.vi"("String"=w322) -> ("boolean"=w321:bool)  [unwired: 6 in, 3 out]
                  n208 = call "CONVERSOR.vi"("String"=w329) -> ("boolean"=w328:bool)  [unwired: 6 in, 3 out]
                  n209 = call "CONVERSOR.vi"("String"=w326) -> ("boolean"=w325:bool)  [unwired: 6 in, 3 out]
                  n210 = call "CONVERSOR.vi"("String"=w318) -> ("float"=w317:dbl)  [unwired: 6 in, 3 out]
                  n211 = call "CONVERSOR.vi"("String"=w315) -> ("float"=w314:dbl)  [unwired: 6 in, 3 out]
                  n212 = local write "SIK-CV-001"(w324) -> ()
                  n213 = local write "SIW-CV-001"(w328) -> ()
                  n214 = case shown="True" TRUE {
                    tunnel: [w411 w430] -> w387
                    tunnel: [w410 w431] -> w386
                    tunnel: w317 -> [_ w431]
                    tunnel: w314 -> [_ w430]
                    frame False {
                      # "Cálculos de valores de velocidade utilizando informações do CLP"
                      # "área"
                      # "área"
                      n215 = local read "Escala de Calibracao - SKM-FI-WF"() -> (w417:cluster{"Escala Max":dbl, "Escala Min":dbl})
                      n216 = Unbundle By Name("Escala de Calibracao - SKM-FI-WF") -> ("Escala Max"=w420:dbl, "Escala Min"=w419:dbl)
                      n217 = Bundle By Name(cluster=w417, "Escala Max"=0.001805556, "Escala Min"=0.0 ("Escala Max")) -> (w418:cluster{"Escala Max":dbl, "Escala Min":dbl})
                      n218 = Divide(x="SKM-FIC-KF_CORIOLI [kg/s]", y="SKM-AI-KF_CORIOLI [kg/m³]") -> (x/y=w429:dbl)
                      n219 = Divide(x=w429, y=0.0005107051557) -> (x/y=w411:dbl)
                      n220 = local write "Escala de Calibracao - SKM-FI-WF"(w418) -> ()
                      n221 = Subtract(x=w420, y=w419) -> (x-y=w421:dbl)
                      n222 = Divide(x=w421, y=4096.0) -> (x/y=w422:dbl)
                      n223 = Multiply(x=w422, y="Entrada - SKM-FI-WF [CLP]") -> (x*y=w423:dbl)
                      n224 = Add(x=w423, y=w419) -> (x+y=w426:dbl)
                      n225 = Divide(x=w426, y=0.0005107051557) -> (x/y=w410:dbl)
                    }
                    frame True {
                      # "devido a mudança do sistema para não ler valores do CLP , e sim de outro PC\nesse CASE deve ser mantido como TRUE até ordens de mudanças"
                    }
                  }
                  n226 = local read "Pfundo corrente"() -> (w224:dbl)
                  n227 = local read "P1 corrente"() -> (w237:dbl)
                  n228 = local read "P2 corrente"() -> (w236:dbl)
                  n229 = local read "P3 corrente"() -> (w235:dbl)
                  n230 = local read "P4 corrente"() -> (w228:dbl)
                  n231 = local read "JW(m/s)"() -> (w215:dbl)
                  n232 = local read "JK(m/s)"() -> (w214:dbl)
                  n233 = call "variação_pressao_adq.vi"("P1(mA)"=w237, "P2(mA)"=w236, "P3(mA)"=w235, "P4(mA)"=w228, "PFUNDO(mA)"=w224, "JW(m/s)"=w215, "JK(m/s)"=w214, "Valores"=w257, "SIK-CV-001"=w324, "SIW-CV-001"=w328) -> ("P12/L12"=w229:dbl, "P34/L34"=w231:dbl, "P23/L23"=w230:dbl, "P2(kPa)"=w218:dbl, "VALOR TEORICO"=w391:dbl, "P3(kPa)"=w217:dbl, "P1(kPa)"=w219:dbl, "P4(kPa)"=w216:dbl, "P1-P2G"=w234:bool, "P2-P3R"=w225:bool, "P2-P3G"=w233:bool, "P1-P2R"=w227:bool, "P3-P4G"=w232:bool, "P3-P4R"=w226:bool, "PFUNDO(kPa)"=w245:dbl)  [unwired: 3 in]
                  n234 = Bundle By Name(cluster="ValoresEnviados", "Pfundo[kPa]"=w245, "DP_21"=w213, "DP_32"=w212, "DP_43"=w211, "DP_4Atm"=w210) -> (w246:T1)
                  n235 = local write "ValoresEnviados"(w246) -> ()
                  n236 = local write "P1-P2 VERDE"(w234) -> ()
                  n237 = local write "P1-P2 RED"(w227) -> ()
                  n238 = local write "P2-P3 VERDE"(w233) -> ()
                  n239 = local write "P2-P3 RED"(w225) -> ()
                  n240 = local write "P3-P4 VERDE"(w232) -> ()
                  n241 = local write "P3-P4 RED"(w226) -> ()
                  n242 = local write "Pfundo(kPa)"(w245) -> ()
                  n243 = local write "P12/L [Pa/m]"(w229) -> ()
                  n244 = local write "P23/L [Pa/m]"(w230) -> ()
                  n245 = local write "P34/L [Pa/m]"(w231) -> ()
                  n246 = local write "P1(kPa)"(w219) -> ()
                  n247 = local write "P2(kPa)"(w218) -> ()
                  n248 = local write "P3(kPa)"(w217) -> ()
                  n249 = local write "P4(kPa)"(w216) -> ()
                  n250 = call "check-up_adq.vi"("JK(m/s)"=w214, "JW(m/s)"=w215, "P4(kPa)"=w216, "P3(kPa)"=w217, "P2(kPa)"=w218, "P1(kPa)"=w219) -> ("OK 2 R"=w220:bool, "OK 2 G"=w221:bool, "OK RED"=w222:bool, "OK G"=w223:bool)  [unwired: 2 in]
                  n251 = local write "OK2 R"(w220) -> ()
                  n252 = local write "Ok"(w223) -> ()
                  n253 = local write "Ok R"(w222) -> ()
                  n254 = local write "OK2"(w221) -> ()
                  n255 = call <vilib>:"DAQmx Start Task.vi"("task/channels in"=w303, "error in"=w302) -> ("task out"=w398:refnum<k21>, "error out"=w397:errorcluster)  [unwired: 12 in]
                  n256 = local write "JW(m/s)"(w386) -> ()
                  n257 = local write "JK(m/s)"(w387) -> ()
                  n258 = local write "Linha de Teste"(w325) -> ()
                  n259 = call-poly <vilib>:"DAQmx Read.vi"("task/channels in"=w398, "number of samples per channel"="Pontos No Gráfico", "error in"=w397) -> ("task out"=w396:refnum<k21>, "data"=w394:dbl[][], "error out"=w395:errorcluster)  [unwired: 10 in]
                  n260 = case shown="True" w325 {
                    tunnel: w391 -> [_ w434]
                    frame False {
                      n261 = local write "Valor Teórico[Pa/m]"(nan) -> ()
                    }
                    frame True {
                      n262 = local write "Valor Teórico[Pa/m]"(w434) -> ()
                    }
                  }
                  n263 = call <vilib>:"DAQmx Stop Task.vi"("task/channels in"=w396, "error in"=w395) -> ("task out"=w301:refnum<k21>, "error out"=w300:errorcluster)  [unwired: 12 in]
                  n264 = for {
                    tunnel: w394 -> [w435] mode=indexing
                    tunnel: [w436] -> w360 mode=indexing
                    n265 = for {
                      tunnel: w435 -> [w439] mode=indexing
                      tunnel: [w437] -> w436 mode=indexing
                      n266 = Multiply(x=w439, y=1000.0) -> (x*y=w437:dbl)
                    }
                  }
                  n267 = local write "SIW-CV-001"(w328) -> ()
                  n268 = local write "SIK-CV-001"(w324) -> ()
                  n269 = local read "Aplicação"() -> (w253:string)
                  n270 = Build Array(w328, w324) -> (w388:bool[])
                  n271 = Boolean Array To Number(Boolean array=w388) -> (number=w390:u32)
                  n272 = local write "Aquisição Automática"(w321) -> ()
                  n273 = Equal?(x=w253, y="Deslocamento_Retirada_por_Baixo") -> (x = y?=w249:bool)
                  n274 = Equal?(x=w253, y="Deslocamento_Retirada_por_Cima") -> (x = y?=w248:bool)
                  n275 = Build Array(w249, w248) -> (w250:bool[])
                  n276 = Boolean Array To Number(Boolean array=w250) -> (number=w247:u32)
                  n277 = case shown="0, Default" w247 {
                    tunnel: w390 -> [_ w400 w406]
                    tunnel: ["No Conf." w401 w405] -> w389
                    frame 0, Default {
                    }
                    frame 1 {
                      n278 = case shown="0, Default" w400 {
                        tunnel: ["No Conf." "C1" "C2"] -> w401
                        frame 0, Default {
                        }
                        frame 1 {
                        }
                        frame 2 {
                        }
                      }
                    }
                    frame 2 {
                      n279 = case shown="0, Default" w406 {
                        tunnel: ["No Conf." "C3" "C4"] -> w405
                        frame 0, Default {
                        }
                        frame 1 {
                        }
                        frame 2 {
                        }
                      }
                    }
                  }
                  "Configuração" <- w389
                  n280 = case shown="True" w321 {
                    frame False {
                    }
                    frame True {
                      # "Caso a válvula de aquisição\nseja acionada, a visualização \ndeve encerrar, para começar\na gravaçaao"
                      n281 = local write "Pontos No Gráfico"(10.0 ("POINTS IN GRAPH")) -> ()
                    }
                  }
                  n282 = Index Array(array=w360, index (row) #1=0 ("index (row)"), index (row) #2=1 ("index (row)"), index (row) #3=2 ("index (row)"), index (row) #4=3 ("index (row)"), index (row) #5=4 ("index (row)"), index (row) #6=5 ("index (row)")) -> (element #1=w352:dbl[], element #2=w351:dbl[], element #3=w350:dbl[], element #4=w349:dbl[], element #5=w348:dbl[], element #6=w347:dbl[])  [unwired: 6 in]
                  n283 = Index Array(array=w360, index (row) #1=7 ("index (row)"), index (row) #2=8 ("index (row)"), index (row) #3=9 ("index (row)"), index (row) #4=10 ("index (row)"), index (row) #5=11 ("index (row)"), index (row) #6=12 ("index (row)")) -> (element #1=w340:dbl[], element #2=w339:dbl[], element #3=w338:dbl[], element #4=w337:dbl[], element #5=w336:dbl[], element #6=w335:dbl[])  [unwired: 6 in]
                  n284 = Index Array(array=w360, index (row)=6) -> (element=w333:dbl[])  [unwired: 1 in]
                  n285 = Build Array(w352, w351, w350, w349, w348, w347, w340, w339, w338, w337, w336, w335, w333) -> (→"Gráfico":dbl[][])
                  n286 = local read "SAIR"() -> (w239:bool)
                  n287 = Index Array(array=w360, index (row) #1=0 ("index (row)"), index (row) #2=1 ("index (row)"), index (row) #3=2 ("index (row)"), index (row) #4=3 ("index (row)"), index (row) #5=4 ("index (row)"), index (row) #6=5 ("index (row)"), index (row) #7=6 ("index (row)"), index (row) #8=7 ("index (row)"), index (row) #9=8 ("index (row)"), index (row) #10=9 ("index (row)"), index (row) #11=10 ("index (row)"), index (row) #12=11 ("index (row)"), index (row) #13=12 ("index (row)")) -> (element #1=w393:dbl[], element #2=w384:dbl[], element #3=w372:dbl[], element #4=w371:dbl[], element #5=w370:dbl[], element #6=w369:dbl[], element #7=w368:dbl[], element #8=w367:dbl[], element #9=w366:dbl[], element #10=w365:dbl[], element #11=w364:dbl[], element #12=w363:dbl[], element #13=w362:dbl[])  [unwired: 13 in]
                  n288 = call-poly <vilib>:"Mean.vi"("X"=w393) -> ("mean"=w258:dbl)  [unwired: 1 out]
                  n289 = call-poly <vilib>:"Mean.vi"("X"=w384) -> ("mean"=w259:dbl)  [unwired: 1 out]
                  n290 = call-poly <vilib>:"Mean.vi"("X"=w372) -> ("mean"=w260:dbl)  [unwired: 1 out]
                  n291 = call-poly <vilib>:"Mean.vi"("X"=w371) -> ("mean"=w261:dbl)  [unwired: 1 out]
                  n292 = call-poly <vilib>:"Mean.vi"("X"=w370) -> ("mean"=w262:dbl)  [unwired: 1 out]
                  n293 = call-poly <vilib>:"Mean.vi"("X"=w369) -> ("mean"=w263:dbl)  [unwired: 1 out]
                  n294 = call-poly <vilib>:"Mean.vi"("X"=w368) -> ("mean"=w264:dbl)  [unwired: 1 out]
                  n295 = call-poly <vilib>:"Mean.vi"("X"=w367) -> ("mean"=w265:dbl)  [unwired: 1 out]
                  n296 = call-poly <vilib>:"Mean.vi"("X"=w366) -> ("mean"=w266:dbl)  [unwired: 1 out]
                  n297 = call-poly <vilib>:"Mean.vi"("X"=w365) -> ("mean"=w267:dbl)  [unwired: 1 out]
                  n298 = call-poly <vilib>:"Mean.vi"("X"=w364) -> ("mean"=w268:dbl)  [unwired: 1 out]
                  n299 = call-poly <vilib>:"Mean.vi"("X"=w363) -> ("mean"=w269:dbl)  [unwired: 1 out]
                  n300 = call-poly <vilib>:"Mean.vi"("X"=w362) -> ("mean"=w270:dbl)  [unwired: 1 out]
                  n301 = local write "C2-M corrente"(w261) -> ()
                  n302 = local write "C1-M corrente"(w258) -> ()
                  n303 = local write "C1-J corrente"(w259) -> ()
                  n304 = local write "P1 corrente"(w260) -> ()
                  n305 = local write "C2-J corrente"(w262) -> ()
                  n306 = local write "P2 corrente"(w263) -> ()
                  n307 = local write "Pfundo corrente"(w264) -> ()
                  n308 = local write "C3-M corrente"(w265) -> ()
                  n309 = local write "C3-J corrente"(w266) -> ()
                  n310 = local write "P3 corrente"(w267) -> ()
                  n311 = local write "C4-M corrente"(w268) -> ()
                  n312 = local write "C4-J corrente"(w269) -> ()
                  n313 = local write "P4 corrente"(w270) -> ()
                  n314 = Multiply(x=w264, y=0.25) -> (x*y=w277:dbl)
                  n315 = Multiply(x=w263, y=0.25) -> (x*y=w278:dbl)
                  n316 = Multiply(x=w268, y=0.25) -> (x*y=w273:dbl)
                  n317 = Multiply(x=w265, y=0.25) -> (x*y=w276:dbl)
                  n318 = Multiply(x=w266, y=0.25) -> (x*y=w275:dbl)
                  n319 = Multiply(x=w267, y=0.25) -> (x*y=w274:dbl)
                  n320 = Multiply(x=w269, y=0.25) -> (x*y=w272:dbl)
                  n321 = Multiply(x=w270, y=0.25) -> (x*y=w271:dbl)
                  n322 = Multiply(x=w261, y=0.25) -> (x*y=w280:dbl)
                  n323 = Multiply(x=w262, y=0.25) -> (x*y=w279:dbl)
                  n324 = Multiply(x=w259, y=0.25) -> (x*y=w282:dbl)
                  n325 = Multiply(x=w260, y=0.25) -> (x*y=w281:dbl)
                  n326 = Multiply(x=w258, y=0.25) -> (x*y=w283:dbl)
                  n327 = local write "C1-M"(w283) -> ()
                  n328 = local write "C1-J"(w282) -> ()
                  n329 = local write "P1"(w281) -> ()
                  n330 = local write "C2-M"(w280) -> ()
                  n331 = local write "C2-J"(w279) -> ()
                  n332 = local write "P2"(w278) -> ()
                  n333 = local write "Pfundo"(w277) -> ()
                  n334 = local write "C3-M"(w276) -> ()
                  n335 = local write "C3-J"(w275) -> ()
                  n336 = local write "P3"(w274) -> ()
                  n337 = local write "C4-M"(w273) -> ()
                  n338 = local write "C4-J"(w272) -> ()
                  n339 = local write "P4"(w271) -> ()
                  "led viewing" <- w241
                  "Visualização" <- w241
                }
                frame 2, 3 {
                  n340 = flat-sequence {
                    tunnel: [w517] -> w449
                    tunnel: [w516] -> w448
                    tunnel: w447 -> [w515]
                    tunnel: w446 -> [w514]
                    tunnel: w445 -> [w513]
                    tunnel: w442 -> [w459]
                    tunnel: [w502] -> w441
                    tunnel: [w501] -> w440
                    tunnel: [w689] -> w443
                    tunnel: [w690] -> w444
                    tunnel: w440 -> [w689]
                    tunnel: w441 -> [w690]
                    frame #0 {
                      w452 = T4."Disabled and Grayed Out" ("Disabled")
                      # "adiciona o índice nome do arquivo"
                      # "Criação e edição dos nomes dos arquivos"
                      # "Aquisição de dados em paralelo da placa NI"
                      n341 = disable-structure shown="Disabled" {
                        disable-tunnel: [w520 _] -> _
                        frame Disabled {
                          n342 = local read "SIK-CV-001"() -> (w521:bool)
                          n343 = local read "SIW-CV-001"() -> (w522:bool)
                          n344 = Build Array(w522, w521) -> (w524:bool[])
                          n345 = Boolean Array To Number(Boolean array=w524) -> (number=w523:u32)
                          n346 = case shown="0, Default" w523 {
                            tunnel: [1 ("mode") 1 ("mode") 2 ("mode")] -> w520
                            frame 0, Default {
                            }
                            frame 1 {
                            }
                            frame 2 {
                            }
                          }
                        }
                        frame Enabled {
                        }
                      }
                      n347 = Current VI's Path() -> (path=w492:path)
                      n348 = Strip Path(path=w492) -> (stripped path=w491:path)  [unwired: 1 out]
                      n349 = property on="pos_processamento" class="Bool"("DisabledEnum"=w452) -> ()  [unwired: 2 in, 2 out]
                      n350 = property on="JW(m/s)" class="DigNum (strict)"("DisabledEnum"=w452) -> ()  [unwired: 2 in, 2 out]
                      n351 = property on="JK(m/s)" class="DigNum (strict)"("DisabledEnum"=w452) -> ()  [unwired: 2 in, 2 out]
                      n352 = property on="Gráfico" class="WFGraph (strict)"("DisabledEnum"=w452) -> ()  [unwired: 2 in, 2 out]
                      n353 = Build Path(base path=w491, name or relative path="PosProcessamento_UDP_NI\\data") -> (appended path=w493:path)
                      n354 = case shown="True" "Retirando agua(?)" {
                        tunnel: [1 ("mode") 2 ("mode")] -> w451
                        frame False {
                        }
                        frame True {
                        }
                      }
                      n355 = local read "JW(m/s)"() -> (w486:dbl)
                      n356 = local read "JG(m/s)"() -> (w482:dbl)
                      n357 = local read "JK(m/s)"() -> (w485:dbl)
                      n358 = Build Array("SIW-CV-001 2", "SIK-CV-001 2") -> (w487:bool[])
                      n359 = Number To Fractional String(number=w486, precision (6)=i16 2) -> (F-format string=w480:string)  [unwired: 2 in]
                      n360 = Number To Fractional String(number=w485, precision (6)=i16 2) -> (F-format string=w479:string)  [unwired: 2 in]
                      n361 = Number To Fractional String(number=w482, precision (6)=i16 2) -> (F-format string=w478:string)  [unwired: 2 in]
                      n362 = local write "Finalizado"(FALSE ("Finalizado")) -> ()
                      n363 = Boolean Array To Number(Boolean array=w487) -> (number=w490:u32)
                      n364 = case shown="2" w490 {
                        tunnel: ["No-Conf." "C1" "C2"] -> w481
                        frame 0, Default {
                        }
                        frame 1 {
                        }
                        frame 2 {
                        }
                      }
                      n365 = local read "Valvulas"() -> (w477:T3)
                      n366 = Current VI's Path() -> (path=w500:path)
                      n367 = Unbundle By Name(w477) -> ("JW"=w476:bool, "JK"=w475:bool, "JG"=w474:bool)
                      n368 = Current VI's Path() -> (path=w509:path)
                      n369 = Strip Path(path=w500) -> (stripped path=w499:path)  [unwired: 1 out]
                      n370 = call "nome_arquivo_adq.vi"("caminho"=w493, "Configuração"=w481, 7:"JW"=w480, 9:"JK"=w479, 11:"JG"=w478, 12:"JW"=w476, 13:"JK"=w475, 14:"JG"=w474) -> ("resulting string"=w461:string)  [unwired: 7 in]
                      n371 = local read "Quantidade de\narquivos adquiridos"() -> (w484:i64)
                      n372 = local read "Quantidade de\narquivos adquiridos"() -> (w456:i64)
                      n373 = Strip Path(path=w509) -> (stripped path=w508:path)  [unwired: 1 out]
                      n374 = Build Path(base path=w499, name or relative path="Aquisicao_UDP_paralelo.vi") -> (appended path=w498:path)
                      n375 = local read "TempoAquisicao"() -> (w458:dbl)
                      n376 = Open VI Reference(type specifier VI Refnum (for type only)=refnum<vi> refnum, vi path=w498, options=128) -> (vi reference=w460:refnum<vi>)  [unwired: 3 in, 1 out]
                      n377 = Build Path(base path=w508, name or relative path="Aquisicao_NI_paralelo.vi") -> (appended path=w507:path)
                      n378 = Open VI Reference(type specifier VI Refnum (for type only)=refnum<vi> refnum, vi path=w507, options=128) -> (vi reference=w506:refnum<vi>, error out=w503:errorcluster)  [unwired: 3 in]
                      n379 = Format Into String(format string="%s%d%s", initial string=w461, "_" ("input 1"), w456, ".UDP" ("substring (\"\")")) -> (resulting string=w463:string)  [unwired: 1 in, 1 out]
                      n380 = local read "Frequência"() -> (w504:dbl)
                      n381 = Increment(x=w484) -> (x+1=w455:i64)
                      n382 = String To Path(string=w463) -> (path=w457:path)
                      n383 = call-by-ref "Start Asynchronous Call"(reference=w460, "file path (dialog if empty)"=w457, "mode"=w451, "Tempo Aquisicao"=w458, "reference in"=w459) -> ()  [unwired: 2 in, 2 out]
                      n384 = Divide(x=w455, y=i64 2) -> (x/y=w453:dbl)
                      n385 = Format Into String(format string="%s%d%s", initial string=w461, "_" ("input 1"), w453, ".NI" ("substring (\"\")")) -> (resulting string=w483:string)  [unwired: 1 in, 1 out]
                      n386 = String To Path(string=w483) -> (path=w466:path)
                      n387 = flat-sequence {
                        frame #0 {
                          n388 = call <vilib>:"Beep.vi"("use system alert? (T)"=FALSE, "duration (msec)"=u32 50, "frequency (Hz)"=u32 528) -> ()  [unwired: 9 in]
                        }
                        frame #1 {
                          # "Aviso sonoro do inicio"
                          n389 = call <vilib>:"Beep.vi"("use system alert? (T)"=FALSE, "duration (msec)"=u32 50, "frequency (Hz)"=u32 665) -> ()  [unwired: 9 in]
                        }
                        frame #2 {
                          n390 = call <vilib>:"Beep.vi"("use system alert? (T)"=FALSE, "duration (msec)"=u32 50, "frequency (Hz)"=u32 790) -> ()  [unwired: 9 in]
                        }
                      }
                      n391 = call-by-ref "Start Asynchronous Call"(reference=w506, error in=w503, "rate"=w504, "Tempo de Aquisição"=w458, "file path (dialog if empty)"=w466, "task/channels in"=refnum<k21> "ADQUIRE" ("DAQmx Task Name")) -> ()  [unwired: 2 in, 5 out]
                      n392 = local write "Quantidade de\narquivos adquiridos"(w453) -> ()
                      n393 = while {
                        tunnel: ["SAIR"] -> w517
                        tunnel: [w545] -> w516
                        tunnel: w515 -> [w550]
                        tunnel: w514 -> [w548]
                        tunnel: w513 -> [w547]
                        tunnel: [errorcluster {"status"=FALSE, "code"=0, "source"=""} ("error out")] -> w502
                        tunnel: [refnum<k21> "ADQUIRE" ("task out")] -> w501
                        i -> [w549]
                        stop <- w551 stop-if-true
                        w541 = TRUE ("adq")
                        n394 = flat-sequence {
                          tunnel: w550 -> [w600]
                          tunnel: w548 -> [w579]
                          tunnel: w547 -> [w564]
                          frame #0 {
                            w556 = TRUE ("visu led")
                            # "aréa de calculo para conversões e analise se os dados encontrados estão dentro de um padrão aceitavel"
                            # "Interpretação dos valores recebidos de outr\nPC e distribuido conforme a necessidade"
                            # "baseado nas configurações de valvulas abertas\né possível saber com qual tipo de configuração \nestá sendo trabalhado"
                            # "SIW-NC-CV-001 05"
                            # "SIK-CV-001 05 04"
                            # "SIT-CV-001 03"
                            # "ADQ 02"
                            # "SPW-WR-VEL 01"
                            # "SPK-WR-VEL 00"
                            n395 = local write "VALORES UDP"(w600) -> ()
                            n396 = Index Array(array=w600, index #1=0 ("index"), index #2=1 ("index"), index #3=2 ("index"), index #4=3 ("index"), index #5=4 ("index"), index #6=5 ("index"), index #7=10 ("index")) -> (element #1=w610:string, element #2=w609:string, element #3=w608:string, element #4=w607:string, element #5=w606:string, element #6=w605:string, element #7=w577:string)
                            n397 = local read "Pfundo corrente"() -> (w625:dbl)
                            n398 = local read "P1 corrente"() -> (w632:dbl)
                            n399 = local read "P2 corrente"() -> (w631:dbl)
                            n400 = local read "P3 corrente"() -> (w630:dbl)
                            n401 = local read "P4 corrente"() -> (w626:dbl)
                            n402 = call "CONVERSOR.vi"("String"=w610) -> ("float"=w580:dbl)  [unwired: 6 in, 3 out]
                            n403 = local write "JK(m/s)"(w580) -> ()
                            n404 = call "CONVERSOR.vi"("String"=w609) -> ("float"=w581:dbl)  [unwired: 6 in, 3 out]
                            n405 = local write "JW(m/s)"(w581) -> ()
                            n406 = call "CONVERSOR.vi"("String"=w608) -> ()  [unwired: 6 in, 4 out]
                            n407 = call "CONVERSOR.vi"("String"=w607) -> ("boolean"=w603:bool)  [unwired: 6 in, 3 out]
                            "Linha de Teste" <- w603
                            n408 = call "CONVERSOR.vi"("String"=w606) -> ("boolean"=w602:bool)  [unwired: 6 in, 3 out]
                            n409 = local write "SIK-CV-001"(w602) -> ()
                            n410 = call "CONVERSOR.vi"("String"=w605) -> ("boolean"=w601:bool)  [unwired: 6 in, 3 out]
                            n411 = local write "SIW-CV-001"(w601) -> ()
                            n412 = call "CONVERSOR.vi"("String"=w577) -> ("boolean"=w576:bool)  [unwired: 6 in, 3 out]
                            n413 = local write "SKS-NC-CV-006"(w576) -> ()
                            n414 = call "variação_pressao_adq.vi"("P1(mA)"=w632, "P2(mA)"=w631, "P3(mA)"=w630, "P4(mA)"=w626, "PFUNDO(mA)"=w625, "JW(m/s)"=w581, "JK(m/s)"=w580, "Valores"=w579, "SIK-CV-001"=w602, "SIW-CV-001"=w601) -> ("P12/L12"=→"P12/L [Pa/m]":dbl, "P34/L34"=→"P34/L [Pa/m]":dbl, "P23/L23"=→"P23/L [Pa/m]":dbl, "P2(kPa)"=w584:dbl, "VALOR TEORICO"=w633:dbl, "P3(kPa)"=w583:dbl, "P1(kPa)"=w585:dbl, "P4(kPa)"=w582:dbl, "P1-P2G"=→"P1-P2 VERDE":bool, "P2-P3R"=→"P2-P3 RED":bool, "P2-P3G"=→"P2-P3 VERDE":bool, "P1-P2R"=→"P1-P2 RED":bool, "P3-P4G"=→"P3-P4 VERDE":bool, "P3-P4R"=→"P3-P4 RED":bool, "PFUNDO(kPa)"=w559:dbl)  [unwired: 3 in]
                            "P4(kPa)" <- w582
                            "P3(kPa)" <- w583
                            "P2(kPa)" <- w584
                            "P1(kPa)" <- w585
                            "Pfundo(kPa)" <- w559
                            n415 = local read "P1(kPa)"() -> (w555:dbl)
                            n416 = local read "P2(kPa)"() -> (w554:dbl)
                            n417 = local read "P3(kPa)"() -> (w553:dbl)
                            n418 = local read "P4(kPa)"() -> (w552:dbl)
                            n419 = local read "ValoresEnviados"() -> (w563:T1)
                            n420 = call "check-up_adq.vi"("JK(m/s)"=w580, "JW(m/s)"=w581, "P4(kPa)"=w582, "P3(kPa)"=w583, "P2(kPa)"=w584, "P1(kPa)"=w585) -> ("OK 2 R"=→"OK2 R":bool, "OK 2 G"=→"OK2":bool, "OK RED"=→"Ok R":bool, "OK G"=→"Ok":bool)  [unwired: 2 in]
                            n421 = Bundle By Name(cluster=w563, "Pfundo[kPa]"=w559, "DP_21"=w555, "DP_32"=w554, "DP_43"=w553, "DP_4Atm"=w552) -> (w565:T1)
                            n422 = case shown="True" w603 {
                              tunnel: w633 -> [_ w668]
                              frame False {
                                n423 = local write "Valor Teórico[Pa/m]"(nan) -> ()
                              }
                              frame True {
                                "Valor Teórico[Pa/m]" <- w668
                              }
                            }
                            n424 = invoke class="VI" method="Ctrl Val.Set"(reference=w564, "Control Name"="ValoresEnviados", "Value"=w563) -> ()  [unwired: 2 in, 5 out]
                            n425 = local write "ValoresEnviados"(w565) -> ()
                            n426 = case shown="False" TRUE {
                              tunnel: [w664 w666] -> w558
                              tunnel: [w649 w665] -> w557
                              tunnel: w581 -> [_ w666]
                              tunnel: w580 -> [_ w665]
                              frame False {
                                n427 = local read "Escala de Calibracao - SKM-FI-WF"() -> (w658:cluster{"Escala Max":dbl, "Escala Min":dbl})
                                n428 = local read "Entrada - SKM-FI-WF [CLP]"() -> (w656:dbl)
                                n429 = local read "SKM-FIC-KF_CORIOLI [kg/s]"() -> (w647:dbl)
                                n430 = local read "SKM-AI-KF_CORIOLI [kg/m³]"() -> (w646:dbl)
                                n431 = local read "Escala de Calibracao - SKM-FI-WF"() -> (w652:cluster{"Escala Max":dbl, "Escala Min":dbl})
                                n432 = Bundle By Name(cluster=w652, "Escala Max"=0.001805556, "Escala Min"=0.0 ("Escala Max")) -> (w653:cluster{"Escala Max":dbl, "Escala Min":dbl})
                                n433 = local write "Escala de Calibracao - SKM-FI-WF"(w653) -> ()
                                n434 = Unbundle By Name(w658) -> ("Escala Max"=w659:dbl, "Escala Min"=w657:dbl)
                                n435 = Divide(x=w647, y=w646) -> (x/y=w648:dbl)
                                n436 = Divide(x=w648, y=0.0005107051557) -> (x/y=w649:dbl)
                                n437 = Subtract(x=w659, y=w657) -> (x-y=w660:dbl)
                                n438 = Divide(x=w660, y=4096.0) -> (x/y=w661:dbl)
                                n439 = Multiply(x=w661, y=w656) -> (x*y=w662:dbl)
                                n440 = Add(x=w662, y=w657) -> (x+y=w663:dbl)
                                n441 = Divide(x=w663, y=0.0005107051557) -> (x/y=w664:dbl)
                              }
                              frame True {
                                # "devido a mudança do sistema para não ler valores do CLP , e sim de outro PC\nesse CASE deve ser mantido como TRUE até ordens de mudanças"
                              }
                            }
                            "JW(m/s)" <- w558
                            "JK(m/s)" <- w557
                            n442 = Index Array(array=w600, index #1=6 ("index"), index #2=7 ("index"), index #3=8 ("index"), index #4=9 ("index")) -> (element #1=w596:string, element #2=w595:string, element #3=w594:string, element #4=w591:string)
                            n443 = call "CONVERSOR.vi"("String"=w596) -> ("float"=w562:dbl)  [unwired: 6 in, 3 out]
                            n444 = call "CONVERSOR.vi"("String"=w595) -> ("float"=w561:dbl)  [unwired: 6 in, 3 out]
                            n445 = call "CONVERSOR.vi"("String"=w594) -> ("float"=w560:dbl)  [unwired: 6 in, 3 out]
                            n446 = call "CONVERSOR.vi"("String"=w591) -> ("float"=w590:dbl)  [unwired: 6 in, 3 out]
                            n447 = local write "JG(m/s)"(w590) -> ()
                            n448 = local write "SKM-FIC-KF-COR"(w561) -> ()
                            n449 = local write "SKM-AI-KF-COR"(w560) -> ()
                            n450 = local write "SKM-FI-WF"(w562) -> ()
                            n451 = local write "SIK-CV-001"(w602) -> ()
                            n452 = local write "SIW-CV-001"(w601) -> ()
                            n453 = local read "Aplicação"() -> (w568:string)
                            n454 = Build Array(w601, w602) -> (w624:bool[])
                            n455 = Boolean Array To Number(Boolean array=w624) -> (number=w570:u32)
                            n456 = for {
                              N: 3000 -> [_]
                              tunnel: [w675] -> _ mode=indexing
                              tunnel: w570 -> [w676]
                              tunnel: [w674] -> _ mode=indexing
                              tunnel: [w673] -> _ mode=indexing
                              tunnel: [w672] -> _ mode=indexing
                              tunnel: w562 -> [w671]
                              tunnel: w561 -> [w670]
                              tunnel: w560 -> [w669]
                              n457 = case shown="0, Default" w676 {
                                tunnel: [w677 w681 w685] -> w675
                                tunnel: [w677 w680 w684] -> w674
                                tunnel: [w677 w679 w683] -> w673
                                tunnel: [w677 w678 w682] -> w672
                                tunnel: w671 -> [_ w680 w684]
                                tunnel: w670 -> [_ w679 w683]
                                tunnel: w669 -> [_ w678 w682]
                                frame 0, Default {
                                w677 = nan
                                }
                                frame 1 {
                                n458 = local read "JW(m/s)"() -> (w681:dbl)
                                }
                                frame 2 {
                                n459 = local read "JK(m/s)"() -> (w685:dbl)
                                }
                              }
                            }
                            n460 = Equal?(x=w568, y="Deslocamento_Retirada_por_Baixo") -> (x = y?=w572:bool)
                            n461 = Equal?(x=w568, y="Deslocamento_Retirada_por_Cima") -> (x = y?=w571:bool)
                            n462 = Build Array(w572, w571) -> (w573:bool[])
                            n463 = Boolean Array To Number(Boolean array=w573) -> (number=w569:u32)
                            n464 = case shown="2" w569 {
                              tunnel: w570 -> [_ w635 w641]
                              tunnel: ["No Conf." w636 w640] -> w567
                              frame 0, Default {
                              }
                              frame 1 {
                                n465 = case shown="1" w635 {
                                tunnel: ["No Conf." "C1" "C2"] -> w636
                                frame 0, Default {
                                }
                                frame 1 {
                                }
                                frame 2 {
                                }
                                }
                              }
                              frame 2 {
                                n466 = case shown="0, Default" w641 {
                                tunnel: ["No Conf." "C3" "C4"] -> w640
                                frame 0, Default {
                                }
                                frame 1 {
                                }
                                frame 2 {
                                }
                                }
                              }
                            }
                            n467 = local write "Configuração"(w567) -> ()
                            n468 = property on="Pontos No Gráfico" class="Knob (strict)"("DisabledEnum"=T4."Disabled and Grayed Out" ("Disabled")) -> ()  [unwired: 2 in, 2 out]
                            n469 = local write "led viewing"(w556) -> ()
                            n470 = local write "Visualização"(w556) -> ()
                          }
                          frame #1 {
                            n471 = Wait (ms)(milliseconds to wait=u32 1000) -> ()  [unwired: 1 out]
                          }
                        }
                        n472 = To Double Precision Float(number=w549) -> (double precision float=w544:dbl)
                        "Timer" <- w544
                        n473 = Greater Or Equal?(x=w544, y="TempoAquisicao") -> (x >= y?=w545:bool)
                        n474 = Compound Arithmetic op=OR(w545, "SAIR") -> (w551:bool)
                        "LED adquiri" <- w541
                        "Aquisição" <- w541
                      }
                    }
                    frame #1 {
                      n475 = flat-sequence {
                        frame #0 {
                          n476 = call <vilib>:"Beep.vi"("use system alert? (T)"=FALSE, "duration (msec)"=u32 50, "frequency (Hz)"=u32 1184) -> ()  [unwired: 9 in]
                        }
                        frame #1 {
                          n477 = Wait (ms)(milliseconds to wait=u32 1) -> ()  [unwired: 1 out]
                        }
                        frame #2 {
                          n478 = call <vilib>:"Beep.vi"("use system alert? (T)"=FALSE, "duration (msec)"=u32 50, "frequency (Hz)"=u32 790) -> ()  [unwired: 9 in]
                        }
                        frame #3 {
                          n479 = Wait (ms)(milliseconds to wait=u32 1) -> ()  [unwired: 1 out]
                        }
                        frame #4 {
                          n480 = call <vilib>:"Beep.vi"("use system alert? (T)"=FALSE, "duration (msec)"=u32 50, "frequency (Hz)"=u32 1056) -> ()  [unwired: 9 in]
                        }
                        frame #5 {
                          "Finalizado" <- TRUE ("Finalizado")
                        }
                      }
                      n481 = local read "Retirando agua(?)"() -> (w688:bool)
                      n482 = Not(x=w688) -> (.not. x?=w687:bool)
                      "retirando agua_indicador" <- w687
                      n483 = local write "Retirando agua(?)"(w687) -> ()
                    }
                  }
                }
              }
              n484 = Compound Arithmetic op=OR(w157, w158) -> (w159:bool)
              n485 = call <vilib>:"DAQmx Clear Task.vi"("task in"=w115, "error in"=w114) -> ("error out"=→"error out":errorcluster)  [unwired: 13 in]
              "DAQmx Task Name" <- w121
            }
            n486 = invoke class="VI" method="Abort VI"(reference=w89) -> ()  [unwired: 2 in, 3 out]
          }
          frame #2 {
            n487 = case shown="False" TRUE {
              frame False {
                # "salva em arquivo TXT tabela de\ndados com o nome ja montado"
                # "adiciona o índice nome do arquivo"
                # "Valores de entrada de velocidades para salvar no nome do arquivo\nVi também recebe o nome da configuração"
                # "Abre o diretório\"DADOS\" para armazenar os dados"
                # "Criação e edição dos nomes dos arquivos"
                n488 = Current VI's Path() -> (path=w775:path)
                n489 = Strip Path(path=w775) -> (stripped path=w774:path)  [unwired: 1 out]
                n490 = Build Path(base path=w774, name or relative path="dados") -> (appended path=w760:path)
                n491 = call <vilib>:"Check if File or Folder Exists.vi"("path"=w760) -> ("file or folder exists?"=w762:bool, "dup path"=w761:path)  [unwired: 8 in, 1 out]
                n492 = case shown="True" w762 {
                  tunnel: w761 -> [w792 w793]
                  tunnel: [w791 w793] -> w759
                  frame False {
                    n493 = Create Folder(path (use dialog)=w792) -> (created path=w791:path)  [unwired: 2 in, 2 out]
                  }
                  frame True {
                  }
                }
                n494 = local read "JW(m/s)"() -> (w786:dbl)
                n495 = local read "JG(m/s)"() -> (w772:dbl)
                n496 = local read "JK(m/s)"() -> (w785:dbl)
                n497 = Build Array("SIW-CV-001", "SIK-CV-001") -> (w787:bool[])
                n498 = Number To Fractional String(number=w786, precision (6)=i16 2) -> (F-format string=w770:string)  [unwired: 2 in]
                n499 = Number To Fractional String(number=w785, precision (6)=i16 2) -> (F-format string=w769:string)  [unwired: 2 in]
                n500 = Number To Fractional String(number=w772, precision (6)=i16 2) -> (F-format string=w768:string)  [unwired: 2 in]
                n501 = Boolean Array To Number(Boolean array=w787) -> (number=w790:u32)
                n502 = case shown="1" w790 {
                  tunnel: ["No-Conf." "C1" "C2"] -> w771
                  frame 0, Default {
                  }
                  frame 1 {
                  }
                  frame 2 {
                  }
                }
                n503 = local read "Valvulas"() -> (w766:T3)
                n504 = Unbundle By Name(w766) -> ("JW"=w765:bool, "JK"=w764:bool, "JG"=w763:bool)
                n505 = call "nome_arquivo_adq.vi"("caminho"=w759, "Configuração"=w771, 7:"JW"=w770, 9:"JK"=w769, 11:"JG"=w768, 12:"JW"=w765, 13:"JK"=w764, 14:"JG"=w763) -> ("resulting string"=w767:string)  [unwired: 7 in]
                n506 = local read "Quantidade de\narquivos adquiridos"() -> (w782:i64)
                n507 = Current VI's Path() -> (path=w757:path)
                n508 = Increment(x=w782) -> (x+1=w776:i64)
                n509 = Format Into String(format string="%s%d%s", initial string=w767, "_" ("input 1"), w776, ".txt" ("substring (\"\")")) -> (resulting string=w778:string)  [unwired: 1 in, 1 out]
                n510 = String To Path(string=w778) -> (path=w777:path)
                n511 = local write "Quantidade de\narquivos adquiridos"(w776) -> ()
                n512 = Strip Path(path=w757) -> (stripped path=w758:path)  [unwired: 1 out]
                n513 = local read "Matriz"() -> (w748:dbl[][])
                n514 = Build Path(base path=w758, name or relative path="titulo.txt") -> (appended path=w755:path)
                n515 = Transpose 2D Array(2D array=w748) -> (transposed array=w753:dbl[][])
                n516 = call-poly <vilib>:"Read Delimited Spreadsheet.vi"("file path (dialog if empty)"=w755) -> ("first row"=w752:string[])  [unwired: 9 in, 5 out]
                n517 = Number To Fractional String(number=w753, precision (6)=i16 4) -> (F-format string=w751:string[][])  [unwired: 2 in]
                n518 = Build Array (concatenate)(w752, w751) -> (w750:string[][])
                n519 = call-poly <vilib>:"Write Delimited Spreadsheet.vi"("file path (dialog if empty)"=w777, "2D data"=w750) -> ()  [unwired: 12 in, 2 out]
              }
              frame True {
                # "Se estiver na posição SAIR, não será gravado arquivo nenhum"
              }
            }
          }
          frame #3 {
            w797 = FALSE ("Visualisa")
            # "botoões paara posição default"
            n520 = flat-sequence {
              frame #0 {
                # "para VI de comunicação com outro PC\nessa VI necessita se parada somento dessa meneira, de outro modo, dará erro"
                n521 = local read "reference out"() -> (w804:refnum<vi>)
                n522 = To Variant(anything=TRUE) -> (Variant=w801:variant)
                n523 = invoke class="VI" method="Ctrl Val.Set"(reference=w804, "Control Name"="STOP", "Value"=w801) -> ()  [unwired: 2 in, 5 out]
                n524 = Wait (ms)(milliseconds to wait=u32 500) -> ()  [unwired: 1 out]
              }
            }
            n525 = global write "comunicacao.vi" "comunicacao"(TRUE ("comunicacao")) -> ()
            n526 = local write "COMEÇAR"(w797) -> ()
            n527 = local write "Visualizar"(w797) -> ()
            n528 = local write "LED adquiri"(w797) -> ()
            n529 = local write "P1-P2 VERDE"(w797) -> ()
            n530 = local write "P1-P2 RED"(w797) -> ()
            n531 = local write "P2-P3 VERDE"(w797) -> ()
            n532 = local write "P2-P3 RED"(w797) -> ()
            n533 = local write "P3-P4 VERDE"(w797) -> ()
            n534 = local write "P3-P4 RED"(w797) -> ()
            n535 = local write "led viewing"(w797) -> ()
            n536 = local write "OK2"(w797) -> ()
            n537 = local write "OK2 R"(w797) -> ()
            n538 = local write "Ok"(w797) -> ()
            n539 = local write "Ok R"(w797) -> ()
            n540 = local write "Aquisição"(w797) -> ()
            n541 = local write "Aquisição Automática"(w797) -> ()
            n542 = local write "Visualização"(w797) -> ()
            n543 = local write "comunica funcionando"(w797) -> ()
            n544 = local read "SAIR"() -> (w799:bool)
          }
        }
      }
    }
    frame #1 {
      # "Como a VI \"abre aplicacção\" é a ultima a ser fechada\napós o termino do addquiri, será aberto ela denovo \npara caso o usurário deseje realizar outra aquisição \ncom outra aplicação, ou alterar alguma configuração"
      # "fecha VI"
      n545 = property class="VI"(error in=w806, "Front Panel.Open"=FALSE ("Front Panel Window:Open")) -> ()  [unwired: 1 in, 2 out]
      n546 = Current VI's Path() -> (path=w813:path)
      n547 = Strip Path(path=w813) -> (stripped path=w807:path)  [unwired: 1 out]
      n548 = Build Path(base path=w807, name or relative path="abre_aplicacao_adq.vi") -> (appended path=w811:path)
      n549 = Open VI Reference(vi path=w811) -> (vi reference=w810:refnum<vi>)  [unwired: 5 in, 1 out]
      n550 = invoke class="VI" method="Run VI"(reference=w810, "Wait until done"=FALSE ("Wait Until Done"), "Auto Dispose Ref"=FALSE ("Auto Dispose Reference")) -> ()  [unwired: 2 in, 5 out]
    }
  }
